vi "COD主界面（列队使用）.vi"() -> (8 "多列列表框":i32(listbox))   [LabVIEW 2016, in "斯坦道CODMn.lvlib"]
uses:
  <vilib>/Analysis/6fits.llb/Curve Fitting Criteria.ctl
  <vilib>/Utility/miscctls.llb/LVPointTypeDef.ctl
  <vilib>/Plasmionique/MB Master/MB_Master_Serial/MB_Master_Serial.lvclass
  D:/Program Files (x86)/National Instruments/LabVIEW 2016/vi.lib/Plasmionique/MB Master/MB_Master/MB_Master.lvclass
  <vilib>/Utility/config.llb/Read Key (Double).vi
  <vilib>/Utility/config.llb/Read Key (Boolean).vi
  <vilib>/Utility/config.llb/Write Key (Double).vi
  <vilib>/Utility/config.llb/Read Key (I32).vi
  <vilib>/Utility/config.llb/Write Key (Boolean).vi
  <vilib>/Utility/config.llb/Write Key (I32).vi
  <vilib>/Waveform/WDTFileIO.llb/Read Waveform from File.vi
  <vilib>/Plasmionique/MB Master/MB Master.lvlib
  <vilib>/ptbypt/NI_PtbyPt.lvlib
  PLC/PLC.lvlib
  <vilib>/Utility/config.llb/NI_LVConfig.lvlib
  <vilib>/Analysis/NI_AALPro.lvlib
panel:
  out "数据时间":string
  out "断电排液标记":bool
  in  "测量模式":T1(ring)
  in  "高切低阈值":dbl
  in  "低切高阈值":dbl
  out "COM":string
  in  "启用5":bool
  in  "校准5":bool
  in  "泵滴定数5":dbl
  in  "浓度5":dbl
  in  "启用4":bool
  in  "校准4":bool
  in  "泵滴定数4":dbl
  in  "浓度4":dbl
  out "波形时间":timestamp
  in  "历史波形":bool
  out "滴定数-ORP值":u16[](array[numeric]) caption="数组"
  in  "关闭 3":bool
  in  "滴定曲线":bool
  out "ORP滴定曲线2":u16[](graph)
  in  "跨度液浓度":dbl
  out "空白测试标记":bool
  out "跨度核查标记":bool
  out "启动选择 2":u16(ring) items=["水样测试", "标样核查", "零点核查", "跨度核查", "空白测试", "加标回收", "平行样", "校零", "校标"]
  in  "量程选择":enum16{"低量程", "高量程", "0-2量程"}(ring)
  in  "手动控制":bool
  in  "选用水样":enum16{"葡萄糖", "草酸钠"}(ring)
  in  "方程系数":cluster{"X^2":dbl, "X":dbl, "b":dbl} {"X^2" format="%#.6g"; "b" format="%#.6g"; "X" format="%#.6g"}
  out "多项式系数1":dbl[](array[numeric]) caption="多项式系数"
  out "XY图":cluster{"X Values":dbl[], "Y Values":dbl[]}[](graph)
  in  "模型":enum32{"线性", "多项式"}(ring)
  out "启动时间":timestamp format="%<%Y/%m/%d %H:%M:%S>T"
  in  "自动切换量程":bool=TRUE
  in  "24H周期设置":bool[](xcontrol)
  in  "关闭 2":bool
  in  "周期设置":bool
  out "文本.文本":string
  out "r^2":dbl format="%.8g"
  out "拟合公式":string
  out "b":dbl format="%#.4g"
  out "K":dbl format="%#.4f"
  out "当前校准":i32
  in  "启用3":bool
  in  "启用2":bool
  in  "启用1":bool
  in  "校准3":bool
  in  "校准2":bool
  in  "校准1":bool
  in  "泵滴定数3":dbl
  in  "泵滴定数2":dbl
  in  "泵滴定数1":dbl
  in  "浓度3":dbl
  in  "浓度2":dbl
  in  "浓度1":dbl
  in  "写入":bool
  out "测量模式数字":i32
  out "零点核查标记":bool
  out "排液故障":bool
  out "进水样超量程":bool
  out "标样核查标记":bool
  out "平行样测量":bool
  out "加标回收测量":bool
  out "质控样测量":bool
  out "待机":bool
  out "校标错误":bool
  out "校零错误":bool
  out "测量错误":bool
  out "草酸钠报警":bool
  out "高锰酸钾报警":bool
  out "加热故障":bool
  out "温控器故障":bool
  out "ORP故障":bool
  out "排液标记":bool
  out "故障标记":bool
  out "校标标记":bool
  out "校零标记":bool
  out "通讯状态":bool
  out "水样测量":bool
  out "读取KB值":bool
  in  "读取":bool
  in  "返回":bool
  in  "校准配置":bool
  in  "修正系数 2":dbl
  in  "浓度 2":dbl
  in  "温度":dbl
  in  "恒温时间":dbl
  in  "基本量程":enum16{"10mg/L", "20mg/L"}(ring)
  in  "水样":dbl
  in  "蒸馏水":dbl
  in  "标液":dbl
  in  "质控样":dbl
  in  "加标回收":dbl
  in  "草酸钠":dbl
  in  "高锰酸钾":dbl
  in  "硫酸":dbl
  in  "零点泵计量数 2":dbl
  in  "标度泵计量数 2":dbl
  out "标度滴定值":dbl
  out "零点滴定值":dbl
  in  "保存":bool
  in  "关闭":bool
  out "测量数据区":T2 {"单位" items=["ug/L", "mg/L", "ppm", "mg/m3", "cm", "ppb", "ug/m3", "%", "nmol/mol", "umol/mol", "MPN/L", "MPN/100ml", "ng/m3", "NTU", "无量纲", "ms/cm", "us/cm", "℃", "mV", "万个/L"]}
  out "仪器时间":timestamp format="%<%Y/%m/%d %H:%M:%S>T"
  out "秒":u16
  out "分":u16
  out "COD浓度（mg/L)":dbl format="%.2g"
  out "进样管":dbl
  out "高锰酸钾":dbl
  out "草酸钠":dbl
  out "硫酸":dbl
  out "ORP显示":dbl
  out "温度":dbl
  out "加热":bool
  out "搅拌":bool
  out "进硫酸":bool
  out "进加标回收样":bool
  out "进质控样":bool
  out "进标液":bool
  out "进蒸馏水":bool
  out "进水样":bool
  out "进草酸钠":bool
  out "进高锰酸钾":bool
  out "定时启动":bool
  in  "启动":bool
  in  "故障清除":bool
  in  "参数配置":bool
  in  "停止":bool
  in  "单步启动":bool
  out "系统时间":timestamp
  in  "时间校准":bool
  in  "枚举":enum16{"读取数据", "写入数据", "读取写入DATABASE", "读取参数"}(ring)
  out "报警簇":T3
  out "Registers":u16[](array[numeric])
  in  "Slave ID":u8=1
  in  "Serial Config":T4={"baud rate (bps)"=115200, "stop bits"=10, "parity"=0, "flow control"=0, "timeout"=1000, "retries"=1} {"stop bits" items=["1.0"=10, "1.5"=15, "2.0"=20]; "flow control" items=["None", "XON/XOFF", "RTS/CTS", "XON/XOFF & RTS/CTS", "DTR/DSR", "XON/XOFF & DTR/DSR"]; "parity" items=["None", "Odd", "Even", "Mark", "Space"]}
  in  "温度 2":dbl
  in  "浓度":dbl
  in  "修正系数":dbl
  in  "标样浓度 2":dbl
  out "模式（受控）":u16
  in  "VISA resource name":refnum<visa-resource-name>="COM4" caption="VISA资源名称"
  # "测量时间："
  # "水样~加标回收"
  # "mV"
  # "℃"
  # "注：遇到加热故障和排液故障时仪器不能正常启动，\n必须排查故障并点击报警清除按钮方可运行。"
  # "mg/L"
  # "校零校标结果"
  # "基本参数设置"
  # "泵计量参数设置"
  # "校零结果："
  # "校零滴定值："
  # "加热恒温温度（℃）："
  # "水样："
  # "高锰酸钾："
  # "校标结果："
  # "标度滴定值："
  # "零点泵计量值："
  # "恒温时间（分钟）："
  # "蒸馏水："
  # "草酸钠："
  # "标度泵计量值："
  # "标准液浓度（mg/L）："
  # "标液："
  # "标样浓度："
  # "硫酸："
  # "修正系数："
  # "质控样："
  # "跨度液浓度："
  # "基本量程（20mg/L可选）："
  # "加标回收样："
  # "是否启用"
  # "泵滴定数"
  # "浓度"
  # "辅\n助\n计\n算\n区"
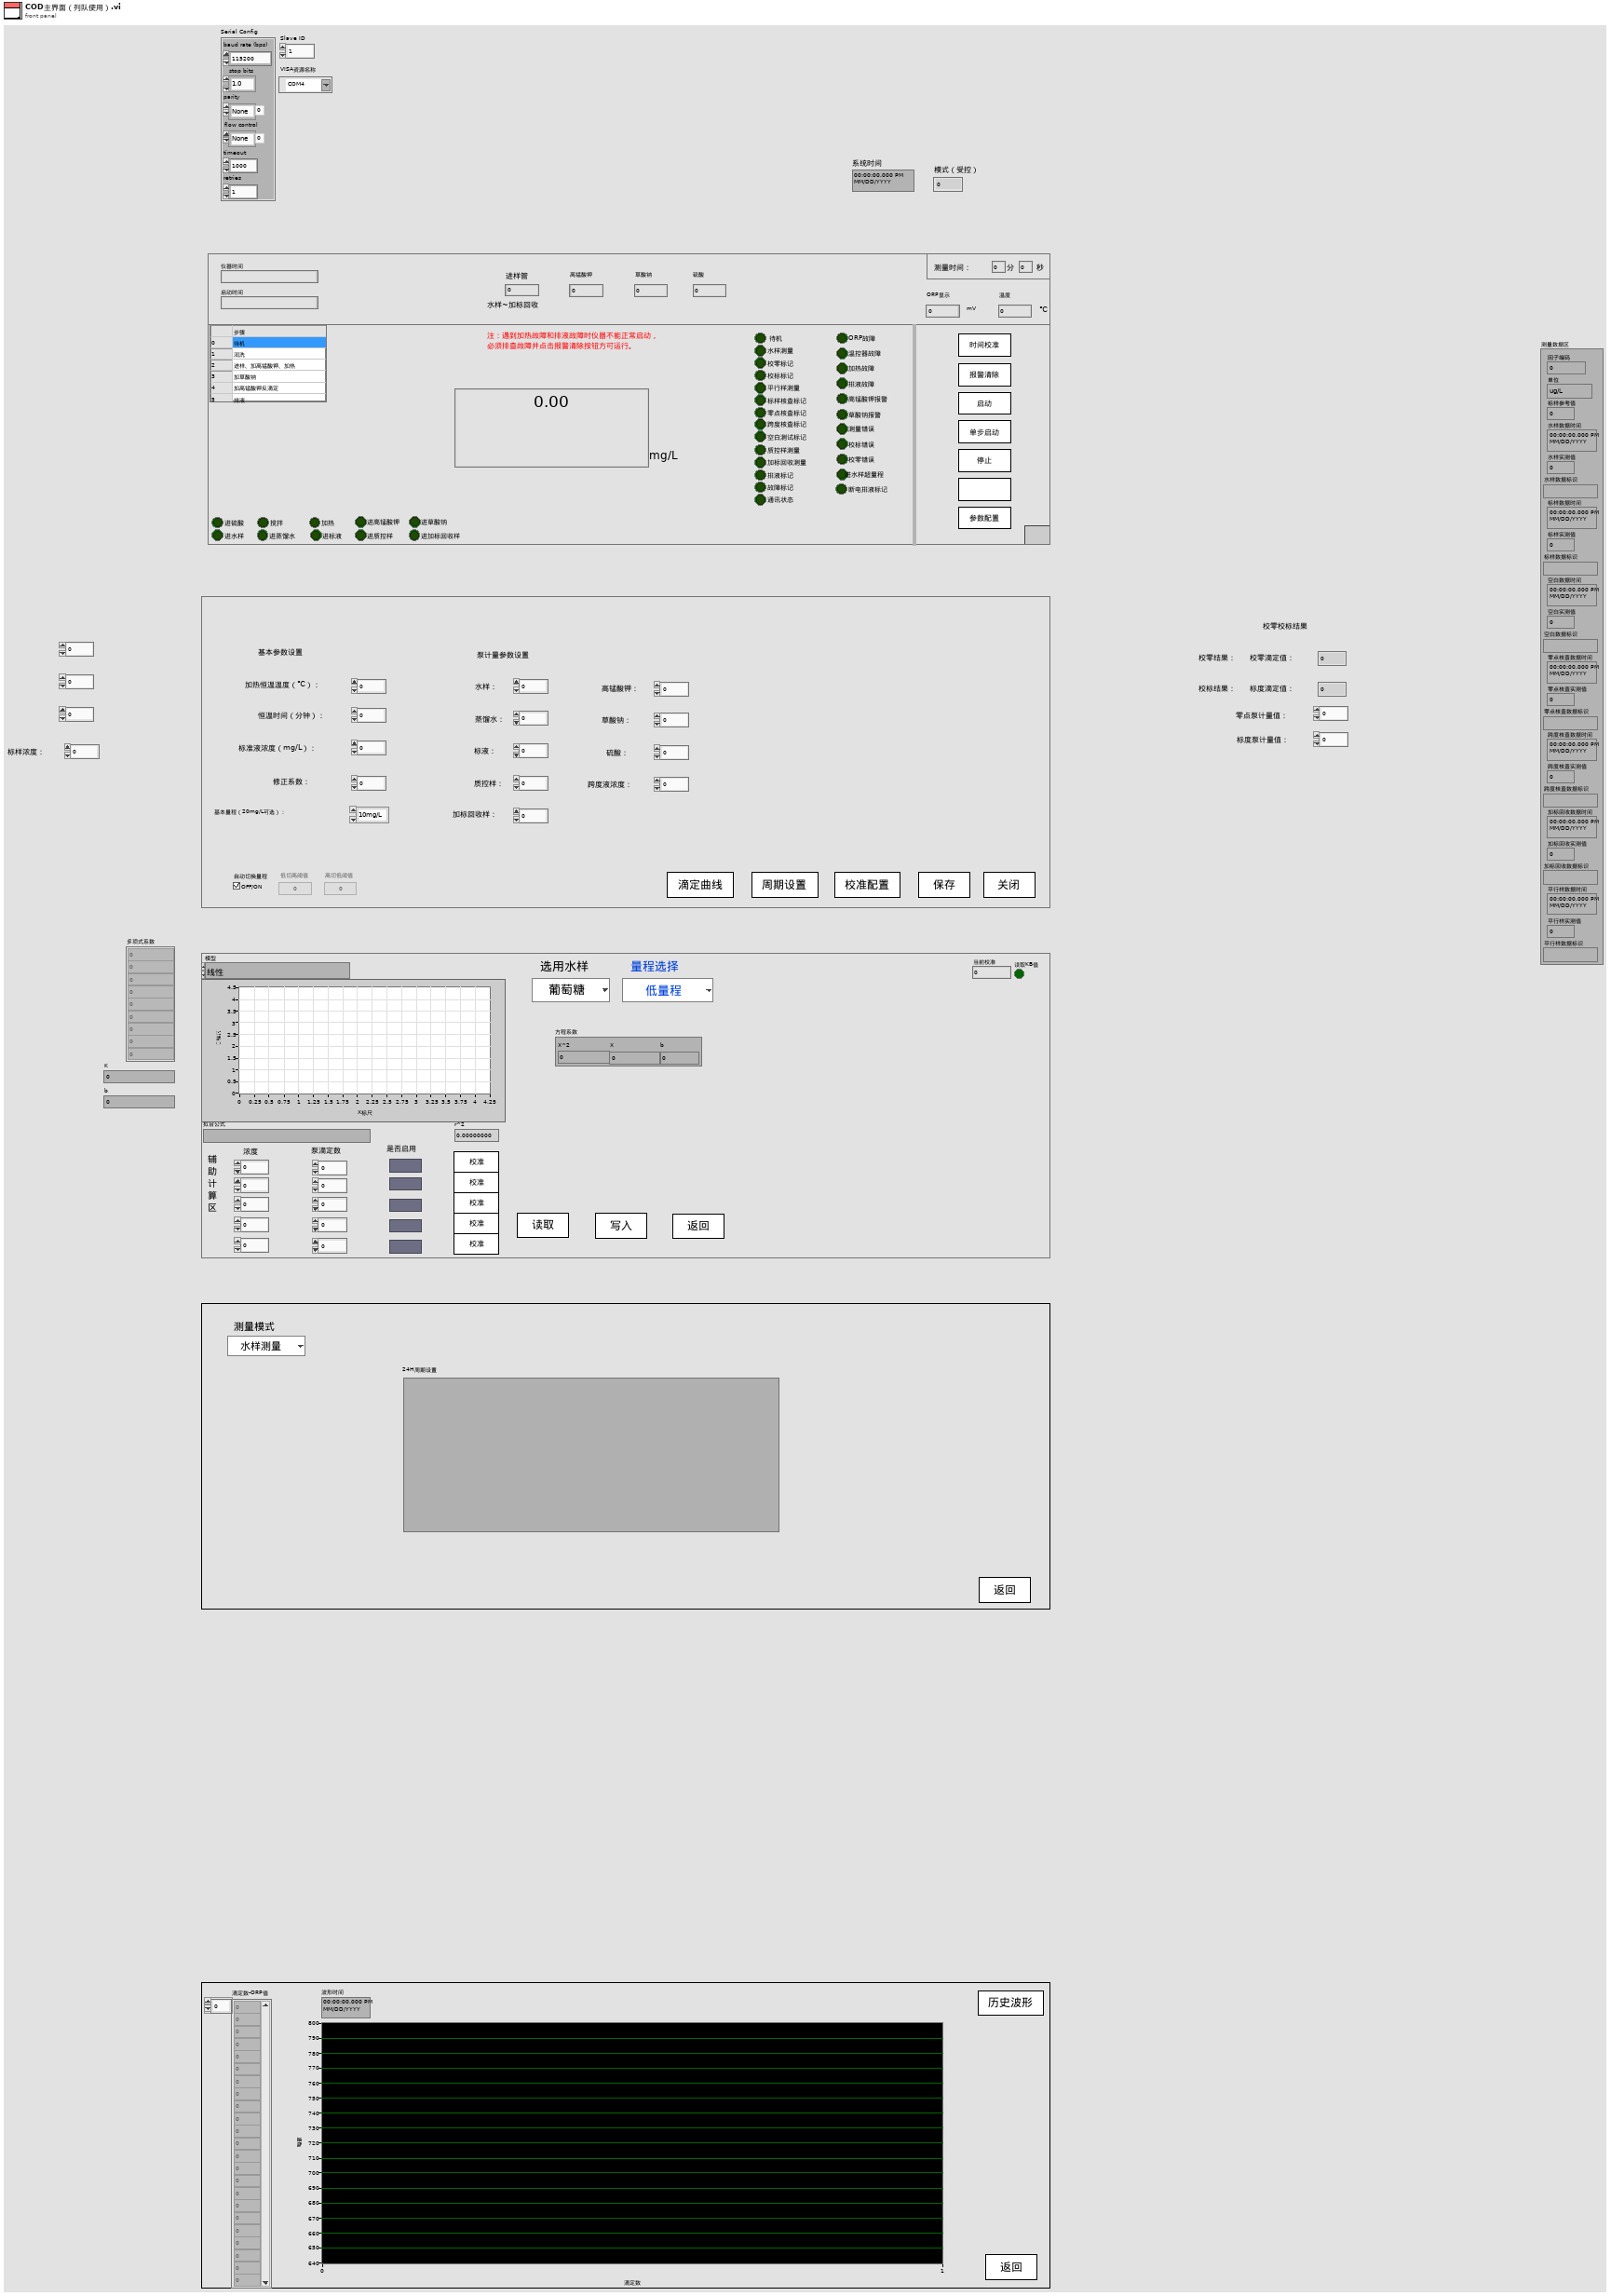
[diagram p1: front panel]
types:
  T1 = enum16{"水样测量", "标样核查", "零点核查", "跨度核查", "空白测试", "加标回收", "平行样", "校零", "校标"}
  T2 = cluster{"因子编码":u32, "单位":u16, "标样参考值":sgl, "水样数据时间":timestamp, "水样实测值":sgl, "水样数据标识":string, "标样数据时间":timestamp, "标样实测值":sgl, "标样数据标识":string, "空白数据时间":timestamp, "空白实测值":sgl, "空白数据标识":string, "零点核查数据时间":timestamp, "零点核查实测值":sgl, "零点核查数据标识":string, "跨度核查数据时间":timestamp, "跨度核查实测值":sgl, "跨度核查数据标识":string, "加标回收数据时间":timestamp, "加标回收实测值":sgl, "加标回收数据标识":string, "平行样数据时间":timestamp, "平行样实测值":sgl, "平行样数据标识":string}
  T3 = cluster{"ORP故障":bool, "温控器故障":bool, "加热故障":bool, "高锰酸钾报警":bool, "草酸钠报警":bool, "测量错误":bool, "校零错误":bool, "校标错误":bool, " 进水样超量程":bool, "排液阀故障":bool}
  T4 = cluster{"baud rate (bps)":u32, "stop bits":u16, "parity":u16, "flow control":u16, "timeout":u32, "retries":i32}
  T5 = cluster{"starting address":u16, "number of holding registers":u16}
  T6 = cluster{"测量模式":enum16{"水样测量", "标样核查", "零点核查", "跨度核查", "空白测试", "加标回收", "平行样", "校零", "校标"}}
  T7 = cluster{"仪器测试类型":enum16{"水样测试", "标样核查", "空白测试", "跨度核查"}, "周期设置类型":enum16{"定点启动", "间隔启动"}, "定时功能启用":bool, "定时间隔":dbl, "24H周期设置":bool[]}
  T8 = typedef "LVDateTimeRec.ctl" = cluster{"秒数的小数部分":dbl, "秒":i32, "分":i32, "时":i32, "日":i32, "月":i32, "年":i32, "天数（周）":i32, "天数（年）":i32, "DST":i32}
  T9 = typedef "LVPointTypeDef.ctl" = cluster{"Horizontal":i16, "Vertical":i16}
  T10 = typedef "NI_LVConfig.lvlib/Config Data RefNum.ctl" = refnum<k1>
  T11 = enum8{"Enabled", "Disabled", "Disabled and Grayed Out"}
  T12 = cluster{"时间标识":timestamp, "参数":string, "日志信息":string, "流程参数":string}
  T13 = cluster{"时间标识":timestamp, "设备":string, "日志信息":string}
  T14 = typedef "NI_AALPro.lvlib/Curve Fitting Criteria.ctl" = u16
  T15 = cluster{"时间标识":timestamp, "设备":string, "日志信息":string, "流程参数":string}
  T16 = cluster{"时间":timestamp, "测量模式":string, "数据类型":string, "检测值":sgl, "单位":string, "数据标识":string, "因子编码":string, "标样参考值":sgl, "ORP-A":sgl, "ORP-B":sgl, "ORP-K":sgl, "COD滴定值":sgl, "高锰酸钾滴定数":sgl, "温度":sgl}
  T17 = cluster{"数组 2[0]":sgl, "数组 2[1]":sgl, "数组 2[2]":sgl, "数组 2[3]":sgl, "数组 2[4]":sgl, "数组 2[5]":sgl, "数组 2[6]":sgl, "数组 2[7]":sgl, "数组 2[8]":sgl}
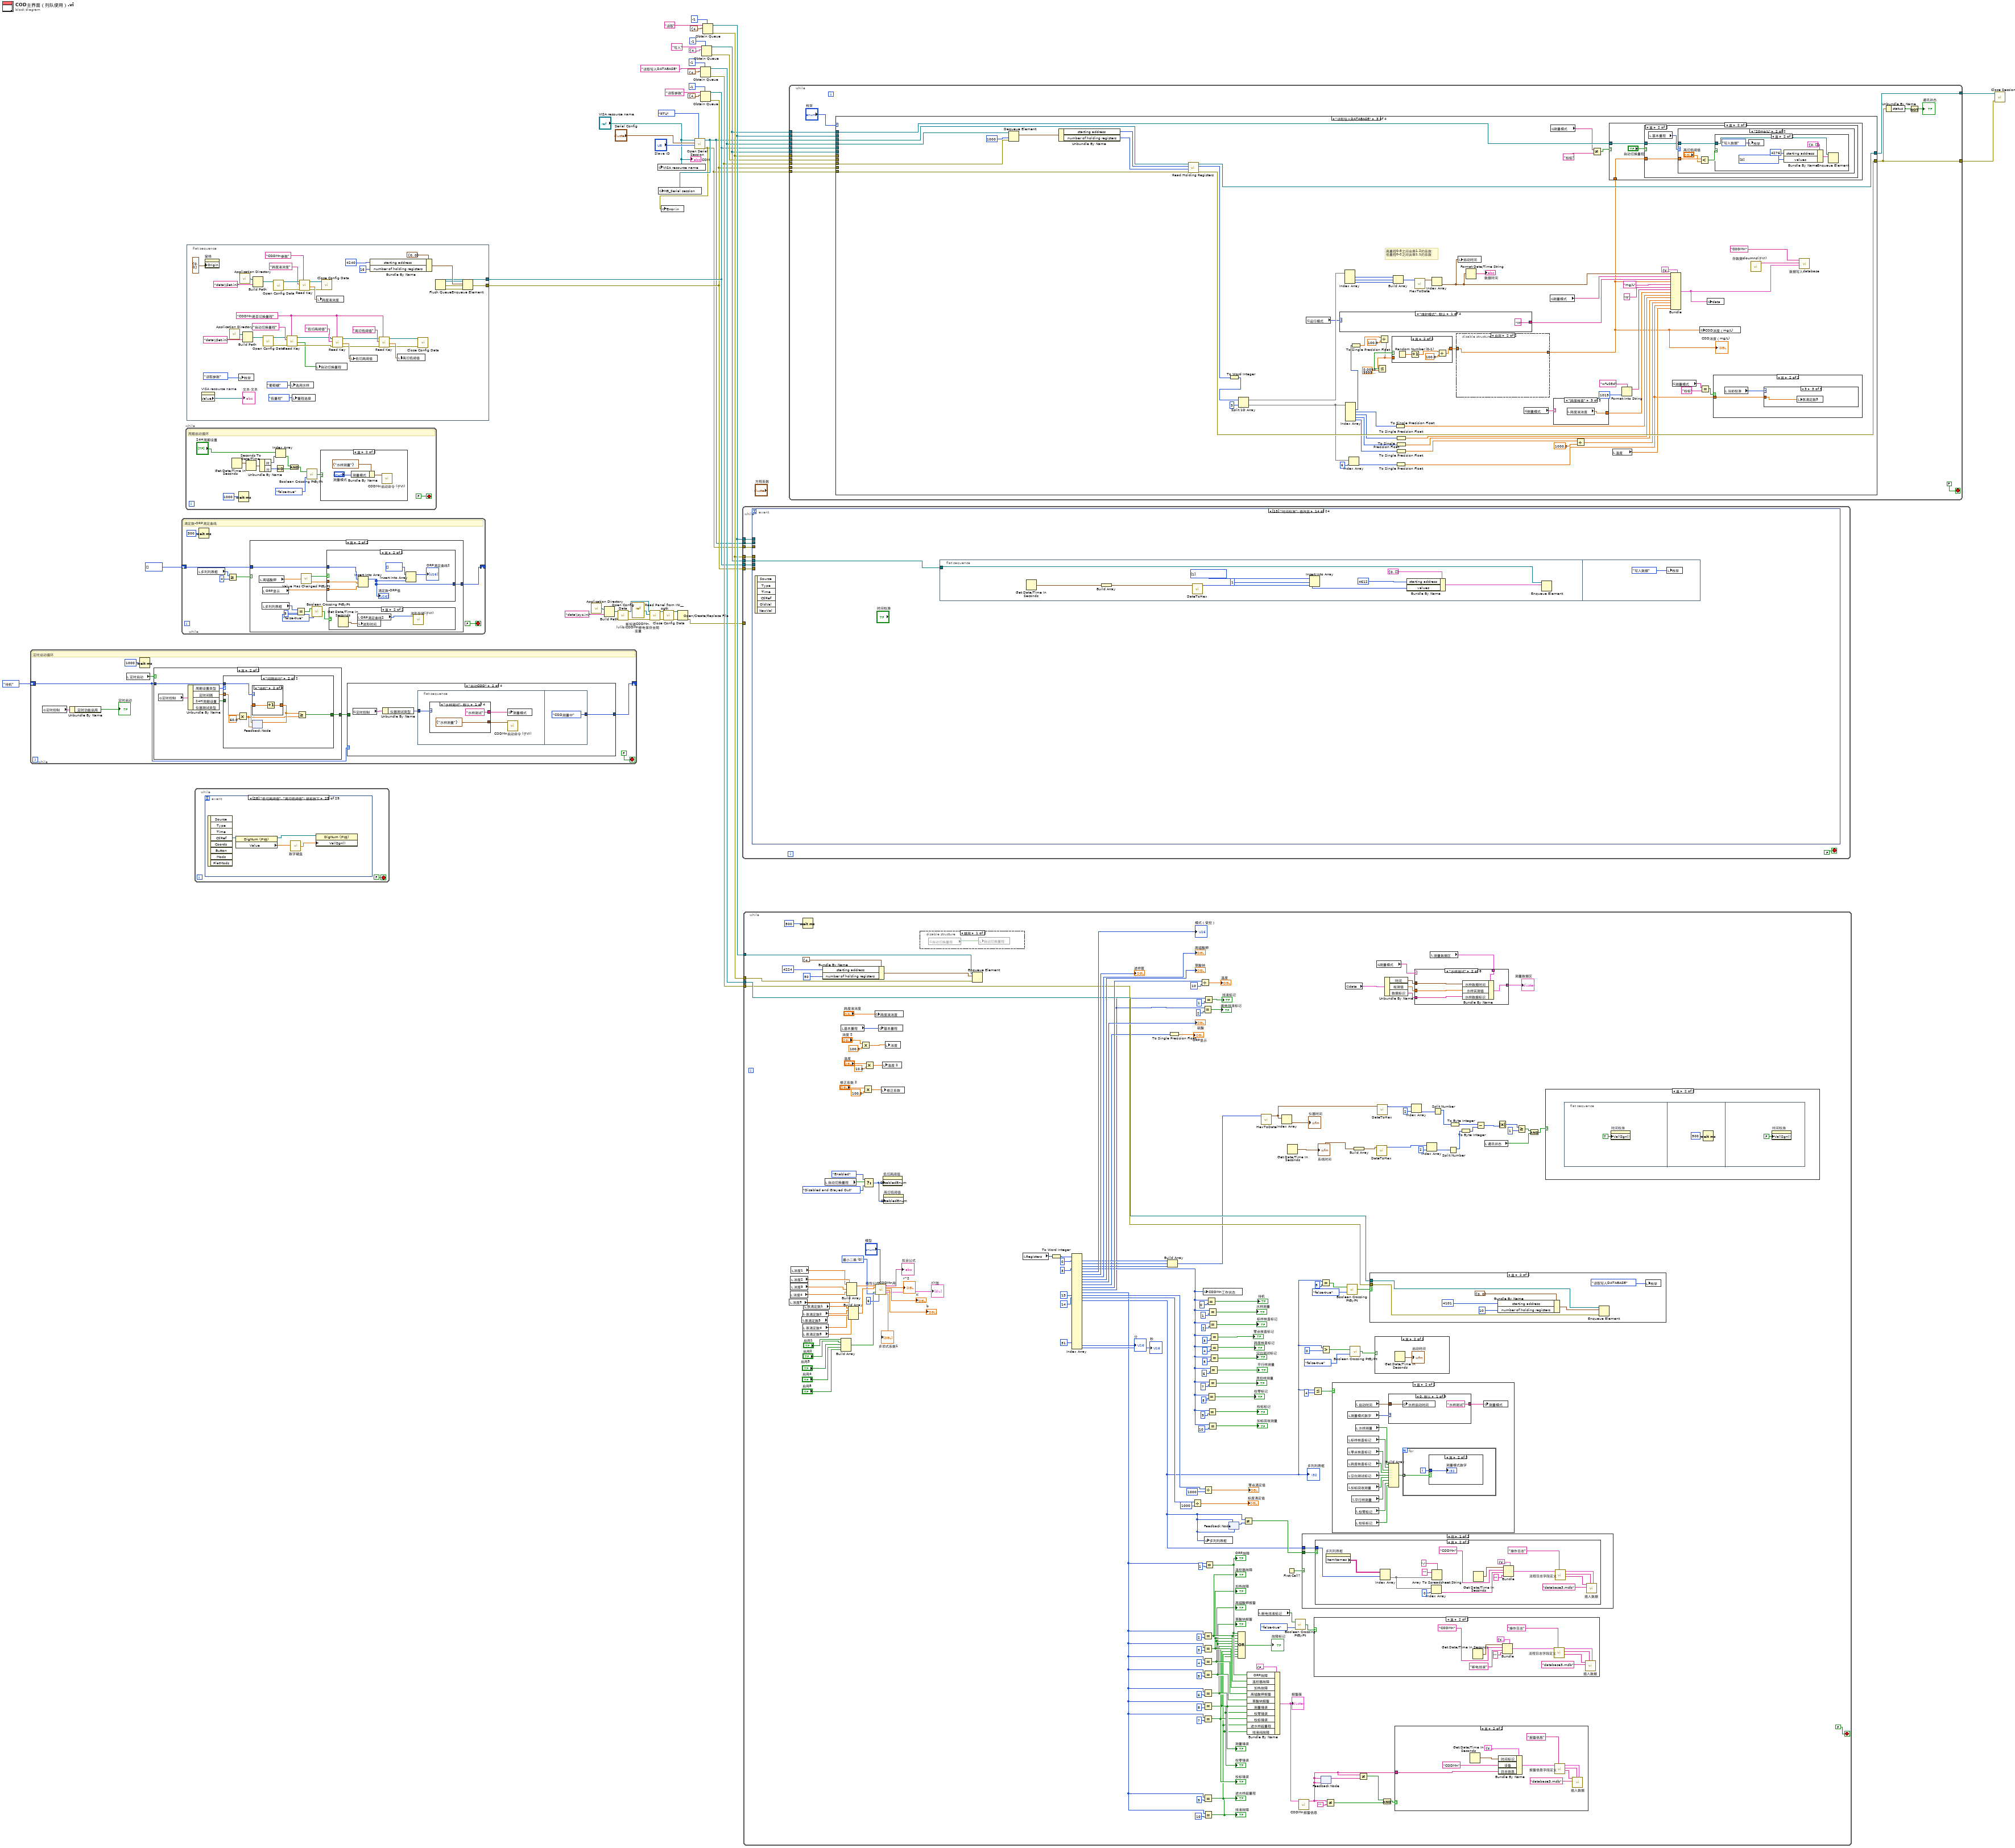
[diagram p0: block diagram]
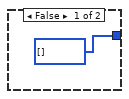
[diagram p2: hidden frame]
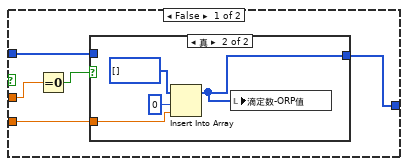
[diagram p4: hidden frame]
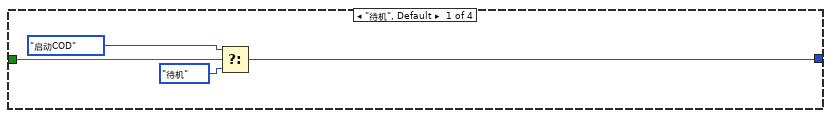
[diagram p7: hidden frame]
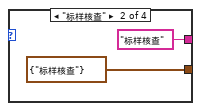
[diagram p8: hidden frame]
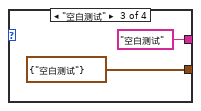
[diagram p9: hidden frame]
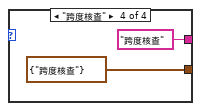
[diagram p10: hidden frame]
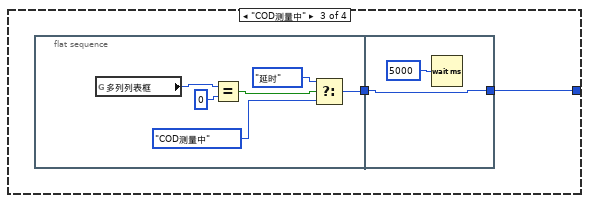
[diagram p11: hidden frame]
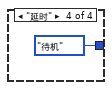
[diagram p12: hidden frame]
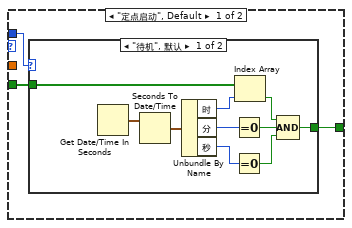
[diagram p14: hidden frame]
diagram:
  n1 = while {
    shift-right: [w47] -> _
    shift-left: enum16{"待机", "启动COD", "COD测量中", "延时"}."待机" -> [w46]
    stop <- FALSE stop-if-true
    # "定时启动循环"
    n2 = global read "CODMn断电保存全局变量.vi" "定时控制"() -> (w43:T7)
    n3 = Unbundle By Name(w43) -> ("定时功能启用"=→"定时启动":bool)
    n4 = local read "定时启动"() -> (w44:bool)
    n5 = Wait (ms)(milliseconds to wait=u32 1000 ("等待时间（毫秒）")) -> ()  [unwired: 1 out]
    n6 = case shown="真" w44 {
      tunnel: w46 -> [_ w82]
      tunnel: [_ w81] -> w45
      frame False {
      }
      frame True {
        n7 = global read "CODMn断电保存全局变量.vi" "定时控制"() -> (w80:T7)
        n8 = Unbundle By Name(w80) -> ("周期设置类型"=w83:enum16{"定点启动", "间隔启动"}, "定时间隔"=w84:dbl, "24H周期设置"=w85:bool[])  [unwired: 1 out]
        n9 = case shown="\"间隔启动\"" w83 {
          tunnel: w84 -> [_ w102]
          tunnel: w85 -> [w88 _]
          tunnel: w82 -> [w86 w105]
          tunnel: [w87 w100] -> w81
          frame "定点启动", Default {
            n10 = case shown="\"待机\", 默认" w86 {
              tunnel: w88 -> [w96 _]
              tunnel: [w89 _] -> w87
              frame "待机", Default {
                n11 = Get Date/Time In Seconds() -> (seconds since 1Jan1904=w98:timestamp)
                n12 = Seconds To Date/Time(time stamp (now)=w98) -> (date time rec=w97:T8)  [unwired: 1 in]
                n13 = Unbundle By Name(w97) -> ("时"=w95:i32, "分"=w93:i32, "秒"=w94:i32)
                n14 = Equal To 0?(x=w93) -> (x = 0?=w91:bool)
                n15 = Equal To 0?(x=w94) -> (x = 0?=w90:bool)
                n16 = Index Array(array=w96, index=w95) -> (element=w92:bool)
                n17 = Compound Arithmetic op=AND ("复合运算")(w92, w91, w90) -> (w89:bool)
              }
              frame "启动COD" {
              }
            }
          }
          frame "间隔启动" {
            n18 = Multiply(x=w102, y=60.0) -> (x*y=w99:dbl)
            n19 = feedback #1(w99) -> (w104:dbl)
            n20 = case shown="\"待机\"" w105 {
              tunnel: w104 -> [_ w107]
              tunnel: [_ w106] -> w103
              frame Default {
              }
              frame "待机" {
                n21 = Increment(x=w107) -> (x+1=w106:dbl)
              }
            }
            n22 = feedback-in #1(w103) -> ()
            n23 = Greater Or Equal?(x=w103, y=w99) -> (x >= y?=w100:bool)
          }
        }
      }
    }
    n24 = case shown="\"启动COD\"" w46 {
      tunnel: [w50 w56 w70 enum16{"待机", "启动COD", "COD测量中", "延时"}."待机"] -> w47
      tunnel: w45 -> [w53 _ _ _]
      frame "待机", Default {
        n25 = Select(t=enum16{"待机", "启动COD", "COD测量中", "延时"}."启动COD", s=w53, f=enum16{"待机", "启动COD", "COD测量中", "延时"}."待机") -> (s? t:f=w50:enum16{"待机", "启动COD", "COD测量中", "延时"})
      }
      frame "启动COD" {
        n26 = global read "CODMn断电保存全局变量.vi" "定时控制"() -> (w54:T7)
        n27 = Unbundle By Name(w54) -> ("仪器测试类型"=w55:enum16{"水样测试", "标样核查", "空白测试", "跨度核查"})
        n28 = flat-sequence {
          tunnel: w55 -> [w59]
          tunnel: [enum16{"待机", "启动COD", "COD测量中", "延时"}."COD测量中"] -> w56
          frame #0 {
            n29 = case shown="\"水样测试\", 默认" w59 {
              tunnel: [T6 {"测量模式"=enum."水样测量"} ("启动测量模式") T6 {"测量模式"=enum."标样核查"} ("启动测量模式") T6 {"测量模式"=enum."空白测试"} ("启动测量模式") T6 {"测量模式"=enum."跨度核查"} ("启动测量模式")] -> w58
              tunnel: ["水样测试" ("测量模式") "标样核查" ("测量模式") "空白测试" ("测量模式") "跨度核查" ("测量模式")] -> w57
              frame "水样测试", Default {
              }
              frame "标样核查" {
              }
              frame "空白测试" {
              }
              frame "跨度核查" {
              }
            }
            n30 = global write "COD测量模式全局.vi" "测量模式"(w57) -> ()
            n31 = call "CODMn启动命令 (子VI).vi"("启动测量模式"=w58) -> ()  [unwired: 11 in]
          }
          frame #1 {
          }
        }
      }
      frame "COD测量中" {
        n32 = flat-sequence {
          tunnel: [w71] -> w69
          tunnel: [w78] -> w70
          tunnel: w69 -> [w78]
          frame #0 {
            n33 = global read "运行时序全局变量.vi" "多列列表框"() -> (w76:i32)
            n34 = Equal?(x=w76, y=0) -> (x = y?=w74:bool)
            n35 = Select(t=enum16{"待机", "启动COD", "COD测量中", "延时"}."延时", s=w74, f=enum16{"待机", "启动COD", "COD测量中", "延时"}."COD测量中") -> (s? t:f=w71:enum16{"待机", "启动COD", "COD测量中", "延时"})
          }
          frame #1 {
            n36 = Wait (ms)(milliseconds to wait=u32 5000 ("等待时间（毫秒）")) -> ()  [unwired: 1 out]
          }
        }
      }
      frame "延时" {
      }
    }
  }
  n37 = while {
    shift-right: [w111] -> _
    shift-left: u16[] [] ("ORP滴定曲线") -> [w112]
    stop <- FALSE stop-if-true
    # "滴定数-ORP滴定曲线"
    n38 = local read "多列列表框"() -> (w110:i32)
    n39 = Wait (ms)(milliseconds to wait=u32 300 ("等待时间（毫秒）")) -> ()  [unwired: 1 out]
    n40 = Greater Or Equal?(x=w110, y=4) -> (x >= y?=w108:bool)
    n41 = case shown="真" w108 {
      tunnel: w112 -> [_ w126]
      tunnel: [u16[] [] ("ORP滴定曲线") w125] -> w111
      frame False {
      }
      frame True {
        n42 = local read "高锰酸钾"() -> (w122:dbl)
        n43 = local read "多列列表框"() -> (w120:i32)
        n44 = local read "ORP显示"() -> (w121:dbl)
        n45 = Equal?(x=w120, y=5) -> (x = y?=w118:bool)
        n46 = call <vilib>:"Value Has Changed PtByPt.vi"("input data point"=w122) -> ("has changed"=w124:bool, "output data point"=w123:dbl)  [unwired: 1 in]
        n47 = call <vilib>:"Boolean Crossing PtByPt.vi"("direction"=enum16{"either", "false-true", "true-false"}."false-true", "input"=w118) -> ("crossing"=w116:bool)  [unwired: 1 in]
        n48 = case shown="真" w124 {
          tunnel: w126 -> [w132 w142]
          tunnel: [w131 w141] -> w125
          tunnel: w123 -> [w133 w140]
          tunnel: w121 -> [w129 w139]
          frame False {
            n49 = Equal To 0?(x=w133) -> (x = 0?=w130:bool)
            n50 = case shown="真" w130 {
              tunnel: [w134 w137] -> w131
              tunnel: w132 -> [w134 _]
              tunnel: w129 -> [_ w136]
              frame False {
              }
              frame True {
                n51 = Insert Into Array(array=u16[] [] ("ORP滴定曲线"), index=0 ("索引"), new element=w136) -> (w137:u16[])
                n52 = local write "滴定数-ORP值"(w137) -> ()
              }
            }
          }
          frame True {
            n53 = Insert Into Array(array=w142, index=w140, new element=w139) -> (w141:u16[])
            "滴定数-ORP值" <- w141
            n54 = Insert Into Array(array=u16[] [] ("ORP滴定曲线"), new element=w141) -> (→"ORP滴定曲线2":u16[])  [unwired: 1 in]
          }
        }
        n55 = case shown="真" w116 {
          frame False {
          }
          frame True {
            n56 = Get Date/Time In Seconds() -> (seconds since 1Jan1904=w127:timestamp)
            n57 = local read "ORP滴定曲线2"() -> (w128:u16[])
            n58 = local write "波形时间"(w127) -> ()
            n59 = call "波形存储(子VI).vi"("ORP滴定曲线"=w128) -> ()  [unwired: 11 in]
          }
        }
      }
    }
  }
  n60 = while "While循环" {
    stop <- FALSE stop-if-true
    # "周期启动循环"
    n61 = Get Date/Time In Seconds() -> (seconds since 1Jan1904=w156:timestamp)
    n62 = Wait (ms)(milliseconds to wait=u32 1000 ("等待时间（毫秒）")) -> ()  [unwired: 1 out]
    n63 = Seconds To Date/Time(time stamp (now)=w156) -> (date time rec=w155:T8)  [unwired: 1 in]
    n64 = Unbundle By Name(w155) -> ("时"=w152:i32, "分"=w154:i32)
    n65 = Equal To 0?(x=w154) -> (x = 0?=w153:bool)
    n66 = Index Array(array="24H周期设置", index=w152) -> (element=w151:bool)
    n67 = And(x=w151, y=w153) -> (x .and. y?=w149:bool)
    n68 = call <vilib>:"Boolean Crossing PtByPt.vi"("direction"=enum16{"either", "false-true", "true-false"}."false-true", "input"=w149) -> ("crossing"=w148:bool)  [unwired: 1 in]
    n69 = case shown="真" w148 {
      frame False {
      }
      frame True {
        n70 = Bundle By Name(cluster=T6 {"测量模式"=enum."水样测量"} ("启动测量模式"), "测量模式"="测量模式") -> (w158:T6)
        n71 = call "CODMn启动命令 (子VI).vi"("启动测量模式"=w158) -> ()  [unwired: 11 in]
      }
    }
  }
  n72 = flat-sequence {
    tunnel: w15 -> [w182]
    tunnel: w14 -> [w181]
    frame #0 {
      w174 = "CODMn是否切换量程" ("key")
      n73 = property on="VISA resource name" class="VISAName"() -> ("Value"=→"文本.文本":refnum<visa-resource-name>)  [unwired: 2 in, 2 out]
      n74 = property on="窗格" class="Pane"("Origin"=T9 {"Horizontal"=0, "Vertical"=0} ("原点")) -> ()  [unwired: 2 in, 2 out]
      n75 = call <vilib>:"Application Directory.vi"() -> ("Application Directory"=w165:path)
      n76 = local write "枚举"(enum16{"读取数据", "写入数据", "读取写入DATABASE", "读取参数"}."读取参数" ("枚举")) -> ()
      n77 = call <vilib>:"Application Directory.vi"() -> ("Application Directory"=w190:path)
      n78 = Build Path(base path=w165, name or relative path="data\\Set.ini" ("名称或相对路径")) -> (appended path=w167:path)
      n79 = Build Path(base path=w190, name or relative path="data\\Set.ini" ("名称或相对路径")) -> (appended path=w192:path)
      n80 = call <vilib>:"Open Config Data.vi"("configuration file path"=w167) -> ("error out"=w164:errorcluster, "refnum"=w163:T10)  [unwired: 8 in, 1 out]
      n81 = call <vilib>:"Open Config Data.vi"("configuration file path"=w192) -> ("error out"=w196:errorcluster, "refnum"=w195:T10)  [unwired: 8 in, 1 out]
      n82 = call-poly <vilib>:"Read Key.vi"("section"=w174, "error in (no error)"=w164, "key"="自动切换量程", "refnum"=w163) -> ("error out"=w171:errorcluster, "value"=w169:bool, "refnum out"=w170:T10)  [unwired: 4 in, 1 out]
      n83 = local write "选用水样"(enum16{"葡萄糖", "草酸钠"}."葡萄糖" ("选用水样")) -> ()
      n84 = local write "量程选择"(enum16{"低量程", "高量程", "0-2量程"}."低量程" ("量程选择")) -> ()
      n85 = call-poly <vilib>:"Read Key.vi"("section"="CODMn参数" ("key"), "error in (no error)"=w196, "key"="跨度液浓度", "refnum"=w195) -> ("error out"=w198:errorcluster, "value"=w199:dbl, "refnum out"=w197:T10)  [unwired: 4 in, 1 out]
      n86 = local write "自动切换量程"(w169) -> ()
      n87 = local write "跨度液浓度"(w199) -> ()
      n88 = call <vilib>:"Close Config Data.vi"("error in (no error)"=w198, "refnum"=w197) -> ()  [unwired: 8 in, 2 out]
      n89 = call-poly <vilib>:"Read Key.vi"("section"=w174, "error in (no error)"=w171, "key"="低切高阈值", "refnum"=w170) -> ("error out"=w173:errorcluster, "value"=w179:dbl, "refnum out"=w172:T10)  [unwired: 4 in, 1 out]
      n90 = local write "低切高阈值"(w179) -> ()
      n91 = Bundle By Name(cluster=T5 {"starting address"=0, "number of holding registers"=0}, "starting address"=u16 4240, "number of holding registers"=u16 16) -> (w189:T5)
      n92 = call-poly <vilib>:"Read Key.vi"("section"=w174, "error in (no error)"=w173, "key"="高切低阈值", "refnum"=w172) -> ("error out"=w176:errorcluster, "value"=w180:dbl, "refnum out"=w175:T10)  [unwired: 4 in, 1 out]
      n93 = local write "高切低阈值"(w180) -> ()
      n94 = call <vilib>:"Close Config Data.vi"("error in (no error)"=w176, "refnum"=w175) -> ()  [unwired: 8 in, 2 out]
      n95 = Flush Queue(queue=w182, error in (no error)=w181) -> (queue out=w185:refnum<queue>, error out=w184:errorcluster)  [unwired: 1 out]
      n96 = Enqueue Element(queue=w185, element=w189, error in (no error)=w184) -> ()  [unwired: 1 in, 3 out]
    }
  }
  n97 = while {
    stop <- FALSE stop-if-true
    n98 = event shown="[28] \"低切高阈值\", \"高切低阈值\": 鼠标按下" {
      selector: _ -> [_ _ _ _ _ _ _ _ _ _ _ _ _ _ _ _ _ _ _ _ _ _ _ _ _ _ _ _ _]
      dyn-events: _ -> [_ _ _ _ _ _ _ _ _ _ _ _ _ _ _ _ _ _ _ _ _ _ _ _ _ _ _ _ _]
      timeout: _ -> [_ _ _ _ _ _ _ _ _ _ _ _ _ _ _ _ _ _ _ _ _ _ _ _ _ _ _ _ _]
      event Timeout {
        n99 = event-data() -> ()  [unwired: 1 in, 3 out]
      }
      event "温度": Mouse Down {
        n100 = event-data() -> ()  [unwired: 1 in, 8 out]
        n101 = local read "温度"() -> (w203:dbl)
        n102 = call "数字键盘.vi"("OldNumber"=w203) -> ("NewNumber"=w202:sgl)
        n103 = local write "温度"(w202) -> ()
      }
      event "恒温时间": Mouse Down {
        n104 = event-data() -> ()  [unwired: 1 in, 8 out]
        n105 = local read "恒温时间"() -> (w204:dbl)
        n106 = call "数字键盘.vi"("OldNumber"=w204) -> ("NewNumber"=w205:sgl)
        n107 = local write "恒温时间"(w205) -> ()
      }
      event "浓度 2": Mouse Down {
        n108 = event-data() -> ()  [unwired: 1 in, 8 out]
        n109 = local read "浓度 2"() -> (w207:dbl)
        n110 = call "数字键盘.vi"("OldNumber"=w207) -> ("NewNumber"=w206:sgl)
        n111 = local write "浓度 2"(w206) -> ()
      }
      event "修正系数 2": Mouse Down {
        n112 = event-data() -> ()  [unwired: 1 in, 8 out]
        n113 = local read "修正系数 2"() -> (w208:dbl)
        n114 = call "数字键盘.vi"("OldNumber"=w208) -> ("NewNumber"=w209:sgl)
        n115 = local write "修正系数 2"(w209) -> ()
      }
      event "水样": Mouse Down {
        n116 = event-data() -> ()  [unwired: 1 in, 8 out]
        n117 = local read "水样"() -> (w210:dbl)
        n118 = call "数字键盘.vi"("OldNumber"=w210) -> ("NewNumber"=w211:sgl)
        n119 = local write "水样"(w211) -> ()
      }
      event "蒸馏水": Mouse Down {
        n120 = event-data() -> ()  [unwired: 1 in, 8 out]
        n121 = local read "蒸馏水"() -> (w212:dbl)
        n122 = call "数字键盘.vi"("OldNumber"=w212) -> ("NewNumber"=w213:sgl)
        n123 = local write "蒸馏水"(w213) -> ()
      }
      event "标液": Mouse Down {
        n124 = event-data() -> ()  [unwired: 1 in, 8 out]
        n125 = local read "标液"() -> (w214:dbl)
        n126 = call "数字键盘.vi"("OldNumber"=w214) -> ("NewNumber"=w215:sgl)
        n127 = local write "标液"(w215) -> ()
      }
      event "质控样": Mouse Down {
        n128 = event-data() -> ()  [unwired: 1 in, 8 out]
        n129 = local read "质控样"() -> (w216:dbl)
        n130 = call "数字键盘.vi"("OldNumber"=w216) -> ("NewNumber"=w217:sgl)
        n131 = local write "质控样"(w217) -> ()
      }
      event "加标回收": Mouse Down {
        n132 = event-data() -> ()  [unwired: 1 in, 8 out]
        n133 = local read "加标回收"() -> (w218:dbl)
        n134 = call "数字键盘.vi"("OldNumber"=w218) -> ("NewNumber"=w219:sgl)
        n135 = local write "加标回收"(w219) -> ()
      }
      event "草酸钠": Mouse Down {
        n136 = event-data() -> ()  [unwired: 1 in, 8 out]
        n137 = local read "草酸钠"() -> (w220:dbl)
        n138 = call "数字键盘.vi"("OldNumber"=w220) -> ("NewNumber"=w221:sgl)
        n139 = local write "草酸钠"(w221) -> ()
      }
      event "高锰酸钾": Mouse Down {
        n140 = event-data() -> ()  [unwired: 1 in, 8 out]
        n141 = local read "高锰酸钾"() -> (w222:dbl)
        n142 = call "数字键盘.vi"("OldNumber"=w222) -> ("NewNumber"=w223:sgl)
        n143 = local write "高锰酸钾"(w223) -> ()
      }
      event "硫酸": Mouse Down {
        n144 = event-data() -> ()  [unwired: 1 in, 8 out]
        n145 = local read "硫酸"() -> (w224:dbl)
        n146 = call "数字键盘.vi"("OldNumber"=w224) -> ("NewNumber"=w225:sgl)
        n147 = local write "硫酸"(w225) -> ()
      }
      event "零点泵计量数 2": Mouse Down {
        n148 = event-data() -> ()  [unwired: 1 in, 8 out]
        n149 = local read "零点泵计量数 2"() -> (w226:dbl)
        n150 = call "数字键盘.vi"("OldNumber"=w226) -> ("NewNumber"=w227:sgl)
        n151 = local write "零点泵计量数 2"(w227) -> ()
      }
      event "标度泵计量数 2": Mouse Down {
        n152 = event-data() -> ()  [unwired: 1 in, 8 out]
        n153 = local read "标度泵计量数 2"() -> (w228:dbl)
        n154 = call "数字键盘.vi"("OldNumber"=w228) -> ("NewNumber"=w229:sgl)
        n155 = local write "标度泵计量数 2"(w229) -> ()
      }
      event "标样浓度 2": Mouse Down {
        n156 = event-data() -> ()  [unwired: 1 in, 8 out]
        n157 = local read "标样浓度 2"() -> (w230:dbl)
        n158 = call "数字键盘.vi"("OldNumber"=w230) -> ("NewNumber"=w231:sgl)
        n159 = local write "标样浓度 2"(w231) -> ()
      }
      event "浓度1": Mouse Down {
        n160 = event-data() -> ()  [unwired: 1 in, 8 out]
        n161 = local read "浓度1"() -> (w233:dbl)
        n162 = call "数字键盘.vi"("OldNumber"=w233) -> ("NewNumber"=w232:sgl)
        n163 = property on="浓度1" class="DigNum (严格)"("Val(Sgnl)"=w232) -> ()  [unwired: 2 in, 2 out]
      }
      event "浓度2": Mouse Down {
        n164 = event-data() -> ()  [unwired: 1 in, 8 out]
        n165 = local read "浓度2"() -> (w235:dbl)
        n166 = call "数字键盘.vi"("OldNumber"=w235) -> ("NewNumber"=w234:sgl)
        n167 = property on="浓度2" class="DigNum (严格)"("Val(Sgnl)"=w234) -> ()  [unwired: 2 in, 2 out]
      }
      event "浓度3": Mouse Down {
        n168 = event-data() -> ()  [unwired: 1 in, 8 out]
        n169 = local read "浓度3"() -> (w237:dbl)
        n170 = call "数字键盘.vi"("OldNumber"=w237) -> ("NewNumber"=w236:sgl)
        n171 = property on="浓度3" class="DigNum (严格)"("Val(Sgnl)"=w236) -> ()  [unwired: 2 in, 2 out]
      }
      event "浓度4": Mouse Down {
        n172 = event-data() -> ()  [unwired: 1 in, 8 out]
        n173 = local read "浓度4"() -> (w239:dbl)
        n174 = call "数字键盘.vi"("OldNumber"=w239) -> ("NewNumber"=w238:sgl)
        n175 = property on="浓度4" class="DigNum (严格)"("Val(Sgnl)"=w238) -> ()  [unwired: 2 in, 2 out]
      }
      event "浓度5": Mouse Down {
        n176 = event-data() -> ()  [unwired: 1 in, 8 out]
        n177 = local read "浓度5"() -> (w241:dbl)
        n178 = call "数字键盘.vi"("OldNumber"=w241) -> ("NewNumber"=w240:sgl)
        n179 = property on="浓度5" class="DigNum (严格)"("Val(Sgnl)"=w240) -> ()  [unwired: 2 in, 2 out]
      }
      event "跨度液浓度": Mouse Down {
        n180 = event-data() -> ()  [unwired: 1 in, 8 out]
        n181 = local read "跨度液浓度"() -> (w243:dbl)
        n182 = call "数字键盘.vi"("OldNumber"=w243) -> ("NewNumber"=w242:sgl)
        n183 = property on="跨度液浓度" class="DigNum (严格)"("Val(Sgnl)"=w242) -> ()  [unwired: 2 in, 2 out]
      }
      event "跨度液浓度": Value Change {
        n184 = event-data() -> ()  [unwired: 1 in, 6 out]
        n185 = call <vilib>:"Application Directory.vi"() -> ("Application Directory"=w247:path)
        n186 = Build Path(base path=w247, name or relative path="data\\Set.ini" ("名称或相对路径")) -> (appended path=w249:path)
        n187 = local read "跨度液浓度"() -> (w244:dbl)
        n188 = call <vilib>:"Open Config Data.vi"("configuration file path"=w249) -> ("error out"=w251:errorcluster, "refnum"=w250:T10)  [unwired: 8 in, 1 out]
        n189 = call-poly <vilib>:"Write Key.vi"("section"="CODMn参数" ("key"), "error in (no error)"=w251, "value"=w244, "key"="跨度液浓度", "refnum"=w250) -> ("error out"=w253:errorcluster, "refnum out"=w252:T10)  [unwired: 4 in, 1 out]
        n190 = call <vilib>:"Close Config Data.vi"("error in (no error)"=w253, "refnum"=w252) -> ()  [unwired: 8 in, 2 out]
      }
      event "泵滴定数1": Mouse Down {
        n191 = event-data() -> ()  [unwired: 1 in, 8 out]
        n192 = local read "泵滴定数1"() -> (w255:dbl)
        n193 = call "数字键盘.vi"("OldNumber"=w255) -> ("NewNumber"=w254:sgl)
        n194 = property on="泵滴定数1" class="DigNum (严格)"("Val(Sgnl)"=w254) -> ()  [unwired: 2 in, 2 out]
      }
      event "泵滴定数2": Mouse Down {
        n195 = event-data() -> ()  [unwired: 1 in, 8 out]
        n196 = local read "泵滴定数2"() -> (w257:dbl)
        n197 = call "数字键盘.vi"("OldNumber"=w257) -> ("NewNumber"=w256:sgl)
        n198 = property on="泵滴定数2" class="DigNum (严格)"("Val(Sgnl)"=w256) -> ()  [unwired: 2 in, 2 out]
      }
      event "泵滴定数3": Mouse Down {
        n199 = event-data() -> ()  [unwired: 1 in, 8 out]
        n200 = local read "泵滴定数3"() -> (w259:dbl)
        n201 = call "数字键盘.vi"("OldNumber"=w259) -> ("NewNumber"=w258:sgl)
        n202 = property on="泵滴定数3" class="DigNum (严格)"("Val(Sgnl)"=w258) -> ()  [unwired: 2 in, 2 out]
      }
      event "泵滴定数4": Mouse Down {
        n203 = event-data() -> ()  [unwired: 1 in, 8 out]
        n204 = local read "泵滴定数4"() -> (w261:dbl)
        n205 = call "数字键盘.vi"("OldNumber"=w261) -> ("NewNumber"=w260:sgl)
        n206 = property on="泵滴定数4" class="DigNum (严格)"("Val(Sgnl)"=w260) -> ()  [unwired: 2 in, 2 out]
      }
      event "泵滴定数5": Mouse Down {
        n207 = event-data() -> ()  [unwired: 1 in, 8 out]
        n208 = local read "泵滴定数5"() -> (w263:dbl)
        n209 = call "数字键盘.vi"("OldNumber"=w263) -> ("NewNumber"=w262:sgl)
        n210 = property on="泵滴定数5" class="DigNum (严格)"("Val(Sgnl)"=w262) -> ()  [unwired: 2 in, 2 out]
      }
      event "低切高阈值", "高切低阈值": Mouse Down {
        n211 = event-data() -> ("CtlRef"=w267:refnum<vi>)  [unwired: 1 in, 7 out]
        n212 = property class="DigNum (严格)"(reference=w267) -> (reference out=w266:refnum<vi>, "Value"=w265:dbl)  [unwired: 1 in, 1 out]
        n213 = call "数字键盘.vi"("OldNumber"=w265) -> ("NewNumber"=w264:sgl)
        n214 = property class="DigNum (严格)"(reference=w266, "Val(Sgnl)"=w264) -> ()  [unwired: 1 in, 2 out]
      }
    }
  }
  n215 = call <vilib>:"Application Directory.vi"() -> ("Application Directory"=w4:path)
  n216 = Build Path(base path=w4, name or relative path="data\\sys.ini" ("名称或相对路径")) -> (appended path=w6:path)
  n217 = call <vilib>:"Open Config Data.vi"("configuration file path"=w6) -> ("error out"=w10:errorcluster, "refnum"=w7:T10)  [unwired: 8 in, 1 out]
  n218 = vi-ref "斯坦道CODMn.lvlib:CODMn断电保存全局变量.vi"() -> (w8:refnum<vi>)
  n219 = call <userlib>:"Read Panel from INI__ogtk.vi"("error in (no error)"=w10, "VI ref"=w8, "refnum"=w7) -> ("error out"=w11:errorcluster, "refnum out"=w9:T10)  [unwired: 7 in]
  n220 = global write "COD浓度全局变量.vi" "VISA resource name"("VISA resource name") -> ()
  n221 = call <vilib>:"Close Config Data.vi"("error in (no error)"=w11, "refnum"=w9) -> ("error out"=w12:errorcluster, "file path"=w13:path)  [unwired: 8 in]
  n222 = Open/Create/Replace File(file path (use dialog)=w13, error in=w12) -> (error out=w3:errorcluster)  [unwired: 4 in, 2 out]
  n223 = call <vilib>:"Open Serial Session.vi"("Mode (RTU)"=enum16{"RTU", "ASCII"}."RTU", "Slave ID"="Slave ID", "Serial Config"="Serial Config", "VISA Resource"="VISA resource name") -> ("Error out"=w1:errorcluster, "MB_Serial session"=w2:refnum<class "MB_Master_Serial.lvclass">)  [unwired: 6 in]
  n224 = global write "COD浓度全局变量.vi" "MB_Serial session"(w2) -> ()
  n225 = global write "COD浓度全局变量.vi" "Error in"(w1) -> ()
  n226 = Obtain Queue(max queue size (-1, unlimited)=-1 ("队列最大值（-1，无限）"), name (unnamed)="读取写入DATABASE" ("名称（未命名）"), element data type=T5 {"starting address"=4224, "number of holding registers"=16}) -> (queue out=w22:refnum<queue>, error out=w21:errorcluster)  [unwired: 2 in, 1 out]
  n227 = Obtain Queue(max queue size (-1, unlimited)=-1 ("队列最大值（-1，无限）"), name (unnamed)="读取参数" ("名称（未命名）"), element data type=T5 {"starting address"=4224, "number of holding registers"=16}) -> (queue out=w15:refnum<queue>, error out=w14:errorcluster)  [unwired: 2 in, 1 out]
  n228 = Obtain Queue(max queue size (-1, unlimited)=-1 ("队列最大值（-1，无限）"), name (unnamed)="写入" ("名称（未命名）"), element data type=cluster{"starting address":u16, "values":u16[]} {"starting address"=4272, "values"=[]}) -> (queue out=w18:refnum<queue>, error out=w20:errorcluster)  [unwired: 2 in, 1 out]
  n229 = Obtain Queue(max queue size (-1, unlimited)=-1 ("队列最大值（-1，无限）"), name (unnamed)="读取" ("名称（未命名）"), element data type=T5 {"starting address"=4224, "number of holding registers"=16}) -> (queue out=w32:refnum<queue>, error out=w31:errorcluster)  [unwired: 2 in, 1 out]
  n230 = while {
    tunnel: w32 -> [w275]
    tunnel: w31 -> [w274]
    tunnel: w18 -> [w273]
    tunnel: w15 -> [w272]
    tunnel: w14 -> [w271]
    tunnel: w2 -> [w269]
    tunnel: w1 -> [w268]
    tunnel: w3 -> [_]
    stop <- FALSE stop-if-true
    n231 = event shown="[13] \"时间校准\": 值改变" {
      selector: _ -> [_ _ _ _ _ _ _ _ _ _ _ _ _ _ _ _ _ _ _ _ _ _ _ _]
      dyn-events: _ -> [_ _ _ _ _ _ _ _ _ _ _ _ _ _ _ _ _ _ _ _ _ _ _ _]
      timeout: _ -> [_ _ _ _ _ _ _ _ _ _ _ _ _ _ _ _ _ _ _ _ _ _ _ _]
      tunnel: w275 -> [_ _ _ _ _ _ _ _ _ _ _ _ _ _ _ _ _ _ _ _ _ _ _ _]
      tunnel: w274 -> [_ _ _ _ _ _ _ _ _ _ _ _ _ _ _ _ _ _ _ _ _ _ _ _]
      tunnel: w273 -> [w283 w316 w353 _ _ w395 _ _ _ _ _ _ _ w755 w769 _ w791 _ _ _ _ w978 _ _]
      tunnel: w272 -> [_ _ _ _ w386 _ _ _ _ _ _ _ _ _ _ _ _ _ _ _ w970 _ _ _]
      tunnel: w271 -> [_ _ _ _ w385 _ _ _ _ _ _ _ _ _ _ _ _ _ _ _ w969 _ _ _]
      tunnel: w269 -> [_ _ _ w359 _ _ _ _ _ _ _ _ w754 _ _ _ _ _ _ _ _ _ _ _]
      tunnel: w268 -> [_ _ _ w358 _ _ _ _ _ _ _ _ w753 _ _ _ _ _ _ _ _ _ _ _]
      event "单步启动": Mouse Down {
        n232 = event-data() -> ()  [unwired: 1 in, 8 out]
        n233 = call "单步启动选择对话框.vi"() -> ("启动选择2"=w276:u16)  [unwired: 10 in, 1 out]
        n234 = case shown="3" w276 {
          tunnel: [u16 4610 ("address") u16 4610 ("address") u16 4610 ("address") u16 4610 ("address") u16 4610 ("address") u16 4610 ("address") u16 4610 ("address") u16 4610 ("address") u16 4610 ("address") u16 4610 ("address") u16 4610 ("address") u16 4610 ("address") u16 4610 ("address")] -> w282
          tunnel: [u16 1 ("address") u16 2 ("address") u16 3 ("address") u16 4 ("address") u16 5 ("address") u16 6 ("address") u16 7 ("address") u16 8 ("address") u16 9 ("holding register value") u16 10 ("holding register value") u16 11 ("holding register value") u16 12 ("address") u16 0 ("address")] -> w279
          frame 0 {
          }
          frame 1 {
          }
          frame 2 {
          }
          frame 3 {
          }
          frame 4 {
          }
          frame 5 {
          }
          frame 6 {
          }
          frame 7 {
          }
          frame 8 {
          }
          frame 9 {
          }
          frame 10 {
          }
          frame 11 {
          }
          frame 12, Default {
          }
        }
        n235 = local write "枚举"(enum16{"读取数据", "写入数据", "读取写入DATABASE", "读取参数"}."写入数据" ("枚举")) -> ()
        n236 = Insert Into Array(array=u16[] [] ("values"), index=0 ("索引"), new element=w279) -> (w278:u16[])
        n237 = Bundle By Name(cluster=cluster{"starting address":u16, "values":u16[]} {"starting address"=0, "values"=[]}, "starting address"=w282, "values"=w278) -> (w284:cluster{"starting address":u16, "values":u16[]})
        n238 = Enqueue Element(queue=w283, element=w284) -> ()  [unwired: 2 in, 3 out]
      }
      event "启动": Mouse Down {
        n239 = event-data() -> ()  [unwired: 1 in, 8 out]
        n240 = flat-sequence {
          tunnel: w316 -> [w319]
          tunnel: [w319] -> w315
          tunnel: [w318] -> w312
          tunnel: w315 -> [w322]
          tunnel: [w322] -> w314
          tunnel: [w320] -> w313
          tunnel: w312 -> [w320]
          tunnel: w314 -> [w324]
          tunnel: w313 -> [w323]
          frame #0 {
            n241 = call "启动测量模式选择对话框.vi"() -> ("启动选择 2"=w318:u16)  [unwired: 11 in]
            "启动选择 2" <- w318
          }
          frame #1 {
            n242 = property on="启动选择 2" class="Ring (严格)"() -> ("RingText.Text"=w321:string)  [unwired: 2 in, 2 out]
            n243 = global write "COD测量模式全局.vi" "测量模式"(w321) -> ()
          }
          frame #2 {
            n244 = case shown="9, 默认" w323 {
              tunnel: [u16 4608 ("address") u16 4608 ("address") u16 4608 ("address") u16 4608 ("address") u16 4608 ("address") u16 4608 ("address") u16 4608 ("address") u16 4608 ("address") u16 4608 ("address") u16 4608 ("address")] -> w325
              tunnel: [u16 1 ("address") u16 2 ("address") u16 3 ("address") u16 4 ("address") u16 5 ("address") u16 7 ("address") u16 6 ("address") u16 8 ("address") u16 9 ("address") u16 0 ("address")] -> w326
              frame 0 {
              }
              frame 1 {
              }
              frame 2 {
              }
              frame 3 {
              }
              frame 4 {
              }
              frame 5 {
              }
              frame 6 {
              }
              frame 7 {
              }
              frame 8 {
              }
              frame 9, Default {
              }
            }
            n245 = Insert Into Array(array=u16[] [] ("values"), index=0 ("索引"), new element=w326) -> (w331:u16[])
            n246 = Bundle By Name(cluster=cluster{"starting address":u16, "values":u16[]} {"starting address"=0, "values"=[]}, "starting address"=w325, "values"=w331) -> (w328:cluster{"starting address":u16, "values":u16[]})
            n247 = Enqueue Element(queue=w324, element=w328) -> ()  [unwired: 2 in, 3 out]
          }
        }
        n248 = local write "枚举"(enum16{"读取数据", "写入数据", "读取写入DATABASE", "读取参数"}."写入数据" ("枚举")) -> ()
      }
      event "停止": Value Change {
        n249 = event-data() -> ()  [unwired: 1 in, 6 out]
        n250 = local write "枚举"(enum16{"读取数据", "写入数据", "读取写入DATABASE", "读取参数"}."写入数据" ("枚举")) -> ()
        n251 = Bundle By Name(cluster=cluster{"starting address":u16, "values":u16[]} {"starting address"=0, "values"=[]}, "starting address"=u16 4608, "values"=u16[] [11]) -> (w355:cluster{"starting address":u16, "values":u16[]})
        n252 = Enqueue Element(queue=w353, element=w355) -> ()  [unwired: 2 in, 3 out]
      }
      event "手动控制": Value Change {
        n253 = event-data() -> ()  [unwired: 1 in, 6 out]
        n254 = call "数字密码键盘.vi"() -> ("NewNumber"=w360:sgl)  [unwired: 1 in]
        n255 = Equal?(x=w360, y=8.0) -> (x = y?=w361:bool)
        n256 = case shown="真" w361 {
          tunnel: w359 -> [_ w365]
          tunnel: w358 -> [_ w364]
          frame False {
            n257 = call "窗口弹出对话框(子VI).vi"("消息"="密码错误") -> ()  [unwired: 10 in, 1 out]
          }
          frame True {
            n258 = call "CODMn手动控制框.vi"("Error in"=w364, "MB_Serial session"=w365) -> ()  [unwired: 10 in]
          }
        }
      }
      event "参数配置": Value Change {
        w372 = "CODMn是否切换量程" ("key")
        n259 = event-data() -> ()  [unwired: 1 in, 6 out]
        n260 = property on="窗格" class="Pane"("Origin"=T9 {"Horizontal"=0, "Vertical"=650} ("原点")) -> ()  [unwired: 2 in, 2 out]
        n261 = Bundle By Name(cluster=T5 {"starting address"=0, "number of holding registers"=0}, "starting address"=u16 4240, "number of holding registers"=u16 16) -> (w393:T5)
        n262 = local write "读取KB值"(FALSE ("读取KB值")) -> ()
        n263 = local write "枚举"(enum16{"读取数据", "写入数据", "读取写入DATABASE", "读取参数"}."读取参数" ("枚举")) -> ()
        n264 = Flush Queue(queue=w386, error in (no error)=w385) -> (queue out=w389:refnum<queue>, error out=w388:errorcluster)  [unwired: 1 out]
        n265 = Enqueue Element(queue=w389, element=w393, error in (no error)=w388) -> ()  [unwired: 1 in, 3 out]
        n266 = call <vilib>:"Application Directory.vi"() -> ("Application Directory"=w381:path)
        n267 = Build Path(base path=w381, name or relative path="data\\Set.ini" ("名称或相对路径")) -> (appended path=w379:path)
        n268 = call <vilib>:"Open Config Data.vi"("configuration file path"=w379) -> ("error out"=w382:errorcluster, "refnum"=w383:T10)  [unwired: 8 in, 1 out]
        n269 = call-poly <vilib>:"Read Key.vi"("section"=w372, "error in (no error)"=w382, "key"="自动切换量程", "refnum"=w383) -> ("error out"=w375:errorcluster, "value"=w377:bool, "refnum out"=w376:T10)  [unwired: 4 in, 1 out]
        n270 = local write "自动切换量程"(w377) -> ()
        n271 = call-poly <vilib>:"Read Key.vi"("section"=w372, "error in (no error)"=w375, "key"="低切高阈值", "refnum"=w376) -> ("error out"=w373:errorcluster, "value"=w367:dbl, "refnum out"=w374:T10)  [unwired: 4 in, 1 out]
        n272 = local write "低切高阈值"(w367) -> ()
        n273 = call-poly <vilib>:"Read Key.vi"("section"=w372, "error in (no error)"=w373, "key"="高切低阈值", "refnum"=w374) -> ("error out"=w370:errorcluster, "value"=w366:dbl, "refnum out"=w371:T10)  [unwired: 4 in, 1 out]
        n274 = local write "高切低阈值"(w366) -> ()
        n275 = call <vilib>:"Close Config Data.vi"("error in (no error)"=w370, "refnum"=w371) -> ()  [unwired: 8 in, 2 out]
      }
      event "保存": Mouse Down {
        n276 = event-data() -> ()  [unwired: 1 in, 8 out]
        n277 = call <vilib>:"Application Directory.vi"() -> ("Application Directory"=w421:path)
        n278 = Build Path(base path=w421, name or relative path="data\\Set.ini" ("名称或相对路径")) -> (appended path=w423:path)
        n279 = local write "枚举"(enum16{"读取数据", "写入数据", "读取写入DATABASE", "读取参数"}."写入数据" ("枚举")) -> ()
        n280 = local read "跨度液浓度"() -> (w418:dbl)
        n281 = call <vilib>:"Open Config Data.vi"("configuration file path"=w423) -> ("error out"=w425:errorcluster, "refnum"=w424:T10)  [unwired: 8 in, 1 out]
        n282 = call-poly <vilib>:"Write Key.vi"("section"="CODMn参数" ("key"), "error in (no error)"=w425, "value"=w418, "key"="跨度液浓度", "refnum"=w424) -> ("error out"=w427:errorcluster, "refnum out"=w426:T10)  [unwired: 4 in, 1 out]
        n283 = call <vilib>:"Close Config Data.vi"("error in (no error)"=w427, "refnum"=w426) -> ()  [unwired: 8 in, 2 out]
        n284 = local write "水样"("水样") -> ()
        n285 = local write "标液"("标液") -> ()
        n286 = local write "硫酸"("硫酸") -> ()
        n287 = local write "恒温时间"("恒温时间") -> ()
        n288 = local write "修正系数"("修正系数") -> ()
        n289 = local write "加标回收"("加标回收") -> ()
        n290 = local write "高锰酸钾"("高锰酸钾") -> ()
        n291 = local write "基本量程"("基本量程") -> ()
        n292 = local write "标样浓度 2"("标样浓度 2") -> ()
        n293 = local write "零点泵计量数 2"("零点泵计量数 2") -> ()
        n294 = local write "标度泵计量数 2"("标度泵计量数 2") -> ()
        n295 = local write "温度 2"("温度 2") -> ()
        n296 = local write "蒸馏水"("蒸馏水") -> ()
        n297 = local write "草酸钠"("草酸钠") -> ()
        n298 = local write "质控样"("质控样") -> ()
        n299 = Build Array("温度 2", "恒温时间", "浓度", "修正系数", "基本量程", "水样", "蒸馏水", "标液", "质控样", "加标回收", "高锰酸钾", "草酸钠", "硫酸", "零点泵计量数 2", "标度泵计量数 2", "标样浓度 2") -> (w410:dbl[])
        n300 = Bundle By Name(cluster=cluster{"starting address":u16, "values":u16[]} {"starting address"=4272, "values"=[]}, "starting address"=u16 4272, "values"=w410) -> (w412:cluster{"starting address":u16, "values":u16[]})
        n301 = Enqueue Element(queue=w395, element=w412, timeout in ms (-1)=1000 ("超时毫秒(-1)")) -> ()  [unwired: 1 in, 3 out]
      }
      event "校准配置": Value Change {
        n302 = event-data() -> ()  [unwired: 1 in, 6 out]
        n303 = property on="窗格" class="Pane"("Origin"=T9 {"Horizontal"=0, "Vertical"=1300} ("原点")) -> ()  [unwired: 2 in, 2 out]
        n304 = call <vilib>:"Application Directory.vi"() -> ("Application Directory"=w478:path)
        n305 = Build Path(base path=w478, name or relative path="data\\Set.ini" ("名称或相对路径")) -> (appended path=w476:path)
        n306 = call <vilib>:"Open Config Data.vi"("configuration file path"=w476) -> ("error out"=w446:errorcluster, "refnum"=w447:T10)  [unwired: 8 in, 1 out]
        n307 = call-poly <vilib>:"Read Key.vi"("section"="CODMn模型选择" ("key"), "error in (no error)"=w446, "key"="线性和多项式", "refnum"=w447) -> ("error out"=w442:errorcluster, "value"=w445:i32, "refnum out"=w443:T10)  [unwired: 4 in, 1 out]
        n308 = local write "模型"(w445) -> ()
        n309 = call-poly <vilib>:"Read Key.vi"("section"="标线选择", "error in (no error)"=w442, "key"="选用水样", "refnum"=w443) -> ("error out"=w440:errorcluster, "value"=w444:i32, "refnum out"=w441:T10)  [unwired: 4 in, 1 out]
        n310 = local write "选用水样"(w444) -> ()
        n311 = local read "量程选择"() -> (w453:enum16{"低量程", "高量程", "0-2量程"})
        n312 = case shown="0, 默认" w444 {
          tunnel: ["葡萄糖标线" ("section") "草酸钠标线" ("section")] -> w452
          frame 0, Default {
          }
          frame 1 {
          }
        }
        n313 = case shown="\"0-2量程\"" w453 {
          tunnel: ["低量程" "高量程" "0-2量程"] -> w451
          frame "低量程", Default {
          }
          frame "高量程" {
          }
          frame "0-2量程" {
          }
        }
        n314 = Concatenate Strings(w452, w451) -> (w450:string)
        n315 = call-poly <vilib>:"Read Key.vi"("section"=w450, "error in (no error)"=w440, "key"="浓度1", "refnum"=w441) -> ("error out"=w482:errorcluster, "value"=w480:dbl, "refnum out"=w481:T10)  [unwired: 4 in, 1 out]
        n316 = local write "浓度1"(w480) -> ()
        n317 = call-poly <vilib>:"Read Key.vi"("section"=w450, "error in (no error)"=w482, "key"="浓度2", "refnum"=w481) -> ("error out"=w496:errorcluster, "value"=w483:dbl, "refnum out"=w495:T10)  [unwired: 4 in, 1 out]
        n318 = local write "浓度2"(w483) -> ()
        n319 = call-poly <vilib>:"Read Key.vi"("section"=w450, "error in (no error)"=w496, "key"="浓度3", "refnum"=w495) -> ("error out"=w497:errorcluster, "value"=w485:dbl, "refnum out"=w494:T10)  [unwired: 4 in, 1 out]
        n320 = local write "浓度3"(w485) -> ()
        n321 = call-poly <vilib>:"Read Key.vi"("section"=w450, "error in (no error)"=w497, "key"="泵滴定数1", "refnum"=w494) -> ("error out"=w498:errorcluster, "value"=w487:dbl, "refnum out"=w493:T10)  [unwired: 4 in, 1 out]
        n322 = local write "泵滴定数1"(w487) -> ()
        n323 = call-poly <vilib>:"Read Key.vi"("section"=w450, "error in (no error)"=w498, "key"="泵滴定数2", "refnum"=w493) -> ("error out"=w492:errorcluster, "value"=w490:dbl, "refnum out"=w499:T10)  [unwired: 4 in, 1 out]
        n324 = local write "泵滴定数2"(w490) -> ()
        n325 = call-poly <vilib>:"Read Key.vi"("section"=w450, "error in (no error)"=w492, "key"="泵滴定数3", "refnum"=w499) -> ("error out"=w504:errorcluster, "value"=w503:dbl, "refnum out"=w500:T10)  [unwired: 4 in, 1 out]
        n326 = local write "泵滴定数3"(w503) -> ()
        n327 = call-poly <vilib>:"Read Key.vi"("section"=w450, "error in (no error)"=w504, "key"="浓度4", "refnum"=w500) -> ("error out"=w505:errorcluster, "value"=w433:dbl, "refnum out"=w501:T10)  [unwired: 4 in, 1 out]
        n328 = local write "浓度4"(w433) -> ()
        n329 = call-poly <vilib>:"Read Key.vi"("section"=w450, "error in (no error)"=w505, "key"="浓度5", "refnum"=w501) -> ("error out"=w438:errorcluster, "value"=w432:dbl, "refnum out"=w439:T10)  [unwired: 4 in, 1 out]
        n330 = local write "浓度5"(w432) -> ()
        n331 = call-poly <vilib>:"Read Key.vi"("section"=w450, "error in (no error)"=w438, "key"="泵滴定数4", "refnum"=w439) -> ("error out"=w506:errorcluster, "value"=w431:dbl, "refnum out"=w502:T10)  [unwired: 4 in, 1 out]
        n332 = local write "泵滴定数4"(w431) -> ()
        n333 = call-poly <vilib>:"Read Key.vi"("section"=w450, "error in (no error)"=w506, "key"="泵滴定数5", "refnum"=w502) -> ("error out"=w436:errorcluster, "value"=w430:dbl, "refnum out"=w437:T10)  [unwired: 4 in, 1 out]
        n334 = local write "泵滴定数5"(w430) -> ()
        n335 = call-poly <vilib>:"Read Key.vi"("section"=w450, "error in (no error)"=w436, "key"="当前选用的校准", "refnum"=w437) -> ("error out"=w472:errorcluster, "value"=w474:i32, "refnum out"=w473:T10)  [unwired: 4 in, 1 out]
        n336 = local write "当前校准"(w474) -> ()
        n337 = call-poly <vilib>:"Read Key.vi"("section"=w450, "error in (no error)"=w472, "key"="启用1", "refnum"=w473) -> ("error out"=w469:errorcluster, "value"=w458:bool, "refnum out"=w470:T10)  [unwired: 4 in, 1 out]
        n338 = local write "启用1"(w458) -> ()
        n339 = call-poly <vilib>:"Read Key.vi"("section"=w450, "error in (no error)"=w469, "key"="启用2", "refnum"=w470) -> ("error out"=w467:errorcluster, "value"=w457:bool, "refnum out"=w468:T10)  [unwired: 4 in, 1 out]
        n340 = local write "启用2"(w457) -> ()
        n341 = call-poly <vilib>:"Read Key.vi"("section"=w450, "error in (no error)"=w467, "key"="启用3", "refnum"=w468) -> ("error out"=w465:errorcluster, "value"=w456:bool, "refnum out"=w466:T10)  [unwired: 4 in, 1 out]
        n342 = local write "启用3"(w456) -> ()
        n343 = call-poly <vilib>:"Read Key.vi"("section"=w450, "error in (no error)"=w465, "key"="启用4", "refnum"=w466) -> ("error out"=w463:errorcluster, "value"=w429:bool, "refnum out"=w464:T10)  [unwired: 4 in, 1 out]
        n344 = local write "启用4"(w429) -> ()
        n345 = call-poly <vilib>:"Read Key.vi"("section"=w450, "error in (no error)"=w463, "key"="启用5", "refnum"=w464) -> ("error out"=w434:errorcluster, "value"=w428:bool, "refnum out"=w435:T10)  [unwired: 4 in, 1 out]
        n346 = local write "启用5"(w428) -> ()
        n347 = call <vilib>:"Close Config Data.vi"("error in (no error)"=w434, "refnum"=w435) -> ()  [unwired: 8 in, 2 out]
      }
      event "选用水样": Value Change {
        (unwired) "浓度6" ("key")
        n348 = event-data() -> ()  [unwired: 1 in, 6 out]
        n349 = property on="窗格" class="Pane"("Origin"=T9 {"Horizontal"=0, "Vertical"=1300} ("原点")) -> ()  [unwired: 2 in, 2 out]
        n350 = local read "量程选择"() -> (w530:enum16{"低量程", "高量程", "0-2量程"})
        n351 = case shown="\"0-2量程\"" w530 {
          tunnel: ["低量程" "高量程" "0-2量程"] -> w531
          frame "低量程", Default {
          }
          frame "高量程" {
          }
          frame "0-2量程" {
          }
        }
        n352 = case shown="\"葡萄糖\", 默认" "选用水样" {
          tunnel: ["葡萄糖标线" ("section") "草酸钠标线" ("section")] -> w532
          frame "葡萄糖", Default {
          }
          frame "草酸钠" {
          }
        }
        n353 = call <vilib>:"Application Directory.vi"() -> ("Application Directory"=w556:path)
        n354 = Build Path(base path=w556, name or relative path="data\\Set.ini" ("名称或相对路径")) -> (appended path=w554:path)
        n355 = call <vilib>:"Open Config Data.vi"("configuration file path"=w554) -> ("error out"=w557:errorcluster, "refnum"=w558:T10)  [unwired: 8 in, 1 out]
        n356 = Concatenate Strings(w532, w531) -> (w529:string)
        n357 = call-poly <vilib>:"Read Key.vi"("section"=w529, "error in (no error)"=w557, "key"="浓度1", "refnum"=w558) -> ("error out"=w562:errorcluster, "value"=w560:dbl, "refnum out"=w561:T10)  [unwired: 4 in, 1 out]
        n358 = local write "浓度1"(w560) -> ()
        n359 = call-poly <vilib>:"Read Key.vi"("section"=w529, "error in (no error)"=w562, "key"="浓度2", "refnum"=w561) -> ("error out"=w576:errorcluster, "value"=w563:dbl, "refnum out"=w575:T10)  [unwired: 4 in, 1 out]
        n360 = local write "浓度2"(w563) -> ()
        n361 = call-poly <vilib>:"Read Key.vi"("section"=w529, "error in (no error)"=w576, "key"="浓度3", "refnum"=w575) -> ("error out"=w577:errorcluster, "value"=w565:dbl, "refnum out"=w574:T10)  [unwired: 4 in, 1 out]
        n362 = local write "浓度3"(w565) -> ()
        n363 = call-poly <vilib>:"Read Key.vi"("section"=w529, "error in (no error)"=w577, "key"="泵滴定数1", "refnum"=w574) -> ("error out"=w578:errorcluster, "value"=w567:dbl, "refnum out"=w573:T10)  [unwired: 4 in, 1 out]
        n364 = local write "泵滴定数1"(w567) -> ()
        n365 = call-poly <vilib>:"Read Key.vi"("section"=w529, "error in (no error)"=w578, "key"="泵滴定数2", "refnum"=w573) -> ("error out"=w572:errorcluster, "value"=w570:dbl, "refnum out"=w579:T10)  [unwired: 4 in, 1 out]
        n366 = local write "泵滴定数2"(w570) -> ()
        n367 = call-poly <vilib>:"Read Key.vi"("section"=w529, "error in (no error)"=w572, "key"="泵滴定数3", "refnum"=w579) -> ("error out"=w584:errorcluster, "value"=w583:dbl, "refnum out"=w580:T10)  [unwired: 4 in, 1 out]
        n368 = local write "泵滴定数3"(w583) -> ()
        n369 = call-poly <vilib>:"Read Key.vi"("section"=w529, "error in (no error)"=w584, "key"="浓度4", "refnum"=w580) -> ("error out"=w585:errorcluster, "value"=w524:dbl, "refnum out"=w581:T10)  [unwired: 4 in, 1 out]
        n370 = local write "浓度4"(w524) -> ()
        n371 = call-poly <vilib>:"Read Key.vi"("section"=w529, "error in (no error)"=w585, "key"="浓度5", "refnum"=w581) -> ("error out"=w527:errorcluster, "value"=w523:dbl, "refnum out"=w528:T10)  [unwired: 4 in, 1 out]
        n372 = local write "浓度5"(w523) -> ()
        n373 = call-poly <vilib>:"Read Key.vi"("section"=w529, "error in (no error)"=w527, "key"="泵滴定数4", "refnum"=w528) -> ("error out"=w586:errorcluster, "value"=w522:dbl, "refnum out"=w582:T10)  [unwired: 4 in, 1 out]
        n374 = local write "泵滴定数4"(w522) -> ()
        n375 = call-poly <vilib>:"Read Key.vi"("section"=w529, "error in (no error)"=w586, "key"="泵滴定数5", "refnum"=w582) -> ("error out"=w525:errorcluster, "value"=w521:dbl, "refnum out"=w526:T10)  [unwired: 4 in, 1 out]
        n376 = local write "泵滴定数5"(w521) -> ()
        n377 = call-poly <vilib>:"Read Key.vi"("section"=w529, "error in (no error)"=w525, "key"="当前选用的校准", "refnum"=w526) -> ("error out"=w550:errorcluster, "value"=w552:i32, "refnum out"=w551:T10)  [unwired: 4 in, 1 out]
        n378 = local write "当前校准"(w552) -> ()
        n379 = call-poly <vilib>:"Read Key.vi"("section"=w529, "error in (no error)"=w550, "key"="启用1", "refnum"=w551) -> ("error out"=w547:errorcluster, "value"=w536:bool, "refnum out"=w548:T10)  [unwired: 4 in, 1 out]
        n380 = local write "启用1"(w536) -> ()
        n381 = call-poly <vilib>:"Read Key.vi"("section"=w529, "error in (no error)"=w547, "key"="启用2", "refnum"=w548) -> ("error out"=w545:errorcluster, "value"=w535:bool, "refnum out"=w546:T10)  [unwired: 4 in, 1 out]
        n382 = local write "启用2"(w535) -> ()
        n383 = call-poly <vilib>:"Read Key.vi"("section"=w529, "error in (no error)"=w545, "key"="启用3", "refnum"=w546) -> ("error out"=w543:errorcluster, "value"=w534:bool, "refnum out"=w544:T10)  [unwired: 4 in, 1 out]
        n384 = local write "启用3"(w534) -> ()
        n385 = call-poly <vilib>:"Read Key.vi"("section"=w529, "error in (no error)"=w543, "key"="启用4", "refnum"=w544) -> ("error out"=w541:errorcluster, "value"=w518:bool, "refnum out"=w542:T10)  [unwired: 4 in, 1 out]
        n386 = local write "启用4"(w518) -> ()
        n387 = call-poly <vilib>:"Read Key.vi"("section"=w529, "error in (no error)"=w541, "key"="启用5", "refnum"=w542) -> ("error out"=w519:errorcluster, "value"=w517:bool, "refnum out"=w520:T10)  [unwired: 4 in, 1 out]
        n388 = local write "启用5"(w517) -> ()
        n389 = call <vilib>:"Close Config Data.vi"("error in (no error)"=w519, "refnum"=w520) -> ()  [unwired: 8 in, 2 out]
      }
      event "量程选择": Value Change {
        n390 = event-data() -> ()  [unwired: 1 in, 6 out]
        n391 = property on="窗格" class="Pane"("Origin"=T9 {"Horizontal"=0, "Vertical"=1300} ("原点")) -> ()  [unwired: 2 in, 2 out]
        n392 = local read "选用水样"() -> (w613:enum16{"葡萄糖", "草酸钠"})
        n393 = case shown="\"葡萄糖\", 默认" w613 {
          tunnel: ["葡萄糖标线" ("section") "草酸钠标线" ("section")] -> w612
          frame "葡萄糖", Default {
          }
          frame "草酸钠" {
          }
        }
        n394 = case shown="\"0-2量程\"" "量程选择" {
          tunnel: ["低量程" "高量程" "0-2量程"] -> w609
          frame "低量程", Default {
          }
          frame "高量程" {
          }
          frame "0-2量程" {
          }
        }
        n395 = call <vilib>:"Application Directory.vi"() -> ("Application Directory"=w636:path)
        n396 = Build Path(base path=w636, name or relative path="data\\Set.ini" ("名称或相对路径")) -> (appended path=w634:path)
        n397 = call <vilib>:"Open Config Data.vi"("configuration file path"=w634) -> ("error out"=w637:errorcluster, "refnum"=w638:T10)  [unwired: 8 in, 1 out]
        n398 = Concatenate Strings(w612, w609) -> (w611:string)
        n399 = call-poly <vilib>:"Read Key.vi"("section"=w611, "error in (no error)"=w637, "key"="浓度1", "refnum"=w638) -> ("error out"=w642:errorcluster, "value"=w640:dbl, "refnum out"=w641:T10)  [unwired: 4 in, 1 out]
        n400 = local write "浓度1"(w640) -> ()
        n401 = call-poly <vilib>:"Read Key.vi"("section"=w611, "error in (no error)"=w642, "key"="浓度2", "refnum"=w641) -> ("error out"=w656:errorcluster, "value"=w643:dbl, "refnum out"=w655:T10)  [unwired: 4 in, 1 out]
        n402 = local write "浓度2"(w643) -> ()
        n403 = call-poly <vilib>:"Read Key.vi"("section"=w611, "error in (no error)"=w656, "key"="浓度3", "refnum"=w655) -> ("error out"=w657:errorcluster, "value"=w645:dbl, "refnum out"=w654:T10)  [unwired: 4 in, 1 out]
        n404 = local write "浓度3"(w645) -> ()
        n405 = call-poly <vilib>:"Read Key.vi"("section"=w611, "error in (no error)"=w657, "key"="泵滴定数1", "refnum"=w654) -> ("error out"=w658:errorcluster, "value"=w647:dbl, "refnum out"=w653:T10)  [unwired: 4 in, 1 out]
        n406 = local write "泵滴定数1"(w647) -> ()
        n407 = call-poly <vilib>:"Read Key.vi"("section"=w611, "error in (no error)"=w658, "key"="泵滴定数2", "refnum"=w653) -> ("error out"=w652:errorcluster, "value"=w650:dbl, "refnum out"=w659:T10)  [unwired: 4 in, 1 out]
        n408 = local write "泵滴定数2"(w650) -> ()
        n409 = call-poly <vilib>:"Read Key.vi"("section"=w611, "error in (no error)"=w652, "key"="泵滴定数3", "refnum"=w659) -> ("error out"=w664:errorcluster, "value"=w663:dbl, "refnum out"=w660:T10)  [unwired: 4 in, 1 out]
        n410 = local write "泵滴定数3"(w663) -> ()
        n411 = call-poly <vilib>:"Read Key.vi"("section"=w611, "error in (no error)"=w664, "key"="浓度4", "refnum"=w660) -> ("error out"=w665:errorcluster, "value"=w600:dbl, "refnum out"=w661:T10)  [unwired: 4 in, 1 out]
        n412 = local write "浓度4"(w600) -> ()
        n413 = call-poly <vilib>:"Read Key.vi"("section"=w611, "error in (no error)"=w665, "key"="浓度5", "refnum"=w661) -> ("error out"=w607:errorcluster, "value"=w599:dbl, "refnum out"=w608:T10)  [unwired: 4 in, 1 out]
        n414 = local write "浓度5"(w599) -> ()
        n415 = call-poly <vilib>:"Read Key.vi"("section"=w611, "error in (no error)"=w607, "key"="泵滴定数4", "refnum"=w608) -> ("error out"=w666:errorcluster, "value"=w598:dbl, "refnum out"=w662:T10)  [unwired: 4 in, 1 out]
        n416 = local write "泵滴定数4"(w598) -> ()
        n417 = call-poly <vilib>:"Read Key.vi"("section"=w611, "error in (no error)"=w666, "key"="泵滴定数5", "refnum"=w662) -> ("error out"=w605:errorcluster, "value"=w597:dbl, "refnum out"=w606:T10)  [unwired: 4 in, 1 out]
        n418 = local write "泵滴定数5"(w597) -> ()
        n419 = call-poly <vilib>:"Read Key.vi"("section"=w611, "error in (no error)"=w605, "key"="当前选用的校准", "refnum"=w606) -> ("error out"=w630:errorcluster, "value"=w632:i32, "refnum out"=w631:T10)  [unwired: 4 in, 1 out]
        n420 = local write "当前校准"(w632) -> ()
        n421 = call-poly <vilib>:"Read Key.vi"("section"=w611, "error in (no error)"=w630, "key"="启用1", "refnum"=w631) -> ("error out"=w627:errorcluster, "value"=w616:bool, "refnum out"=w628:T10)  [unwired: 4 in, 1 out]
        n422 = local write "启用1"(w616) -> ()
        n423 = call-poly <vilib>:"Read Key.vi"("section"=w611, "error in (no error)"=w627, "key"="启用2", "refnum"=w628) -> ("error out"=w625:errorcluster, "value"=w615:bool, "refnum out"=w626:T10)  [unwired: 4 in, 1 out]
        n424 = local write "启用2"(w615) -> ()
        n425 = call-poly <vilib>:"Read Key.vi"("section"=w611, "error in (no error)"=w625, "key"="启用3", "refnum"=w626) -> ("error out"=w623:errorcluster, "value"=w614:bool, "refnum out"=w624:T10)  [unwired: 4 in, 1 out]
        n426 = local write "启用3"(w614) -> ()
        n427 = call-poly <vilib>:"Read Key.vi"("section"=w611, "error in (no error)"=w623, "key"="启用4", "refnum"=w624) -> ("error out"=w621:errorcluster, "value"=w602:bool, "refnum out"=w622:T10)  [unwired: 4 in, 1 out]
        n428 = local write "启用4"(w602) -> ()
        n429 = call-poly <vilib>:"Read Key.vi"("section"=w611, "error in (no error)"=w621, "key"="启用5", "refnum"=w622) -> ("error out"=w603:errorcluster, "value"=w601:bool, "refnum out"=w604:T10)  [unwired: 4 in, 1 out]
        n430 = local write "启用5"(w601) -> ()
        n431 = call <vilib>:"Close Config Data.vi"("error in (no error)"=w603, "refnum"=w604) -> ()  [unwired: 8 in, 2 out]
      }
      event "周期设置": Value Change {
        n432 = event-data() -> ()  [unwired: 1 in, 6 out]
        n433 = call "数字密码键盘.vi"() -> ("NewNumber"=w677:sgl)  [unwired: 1 in]
        n434 = Equal?(x=w677, y=8.0) -> (x = y?=w678:bool)
        n435 = case shown="真" w678 {
          frame False {
            n436 = call "窗口弹出对话框(子VI).vi"("消息"="密码错误") -> ()  [unwired: 10 in, 1 out]
          }
          frame True {
            n437 = call "窗口弹出对话框(子VI).vi"("消息"="登录成功") -> ("true"=w681:bool)  [unwired: 10 in]
            n438 = case shown="真" w681 {
              frame False {
              }
              frame True {
                n439 = property on="窗格" class="Pane"("Origin"=T9 {"Horizontal"=0, "Vertical"=1950} ("原点")) -> ()  [unwired: 2 in, 2 out]
              }
            }
          }
        }
      }
      event "返回": Value Change {
        (unwired) "泵滴定数6" ("key")
        w697 = "CODMn" ("section")
        n440 = event-data() -> ()  [unwired: 1 in, 6 out]
        n441 = property on="窗格" class="Pane"("Origin"=T9 {"Horizontal"=0, "Vertical"=0} ("原点")) -> ()  [unwired: 2 in, 2 out]
        n442 = call <vilib>:"Application Directory.vi"() -> ("Application Directory"=w750:path)
        n443 = Build Path(base path=w750, name or relative path="data\\Set.ini" ("名称或相对路径")) -> (appended path=w748:path)
        n444 = local write "读取KB值"(FALSE ("读取KB值")) -> ()
        n445 = call <vilib>:"Open Config Data.vi"("configuration file path"=w748) -> ("error out"=w746:errorcluster, "refnum"=w747:T10)  [unwired: 8 in, 1 out]
        n446 = local read "浓度1"() -> (w744:dbl)
        n447 = local read "浓度2"() -> (w728:dbl)
        n448 = call-poly <vilib>:"Write Key.vi"("section"=w697, "error in (no error)"=w746, "value"=w744, "key"="浓度1", "refnum"=w747) -> ("error out"=w743:errorcluster, "refnum out"=w742:T10)  [unwired: 4 in, 1 out]
        n449 = local read "浓度3"() -> (w724:dbl)
        n450 = call-poly <vilib>:"Write Key.vi"("section"=w697, "error in (no error)"=w743, "value"=w728, "key"="浓度2", "refnum"=w742) -> ("error out"=w741:errorcluster, "refnum out"=w740:T10)  [unwired: 4 in, 1 out]
        n451 = local read "泵滴定数1"() -> (w722:dbl)
        n452 = call-poly <vilib>:"Write Key.vi"("section"=w697, "error in (no error)"=w741, "value"=w724, "key"="浓度3", "refnum"=w740) -> ("error out"=w739:errorcluster, "refnum out"=w738:T10)  [unwired: 4 in, 1 out]
        n453 = call-poly <vilib>:"Write Key.vi"("section"=w697, "error in (no error)"=w739, "value"=w722, "key"="泵滴定数1", "refnum"=w738) -> ("error out"=w737:errorcluster, "refnum out"=w736:T10)  [unwired: 4 in, 1 out]
        n454 = local read "泵滴定数2"() -> (w720:dbl)
        n455 = call-poly <vilib>:"Write Key.vi"("section"=w697, "error in (no error)"=w737, "value"=w720, "key"="泵滴定数2", "refnum"=w736) -> ("error out"=w735:errorcluster, "refnum out"=w734:T10)  [unwired: 4 in, 1 out]
        n456 = local read "泵滴定数3"() -> (w718:dbl)
        n457 = local read "浓度4"() -> (w685:dbl)
        n458 = call-poly <vilib>:"Write Key.vi"("section"=w697, "error in (no error)"=w735, "value"=w718, "key"="泵滴定数3", "refnum"=w734) -> ("error out"=w733:errorcluster, "refnum out"=w732:T10)  [unwired: 4 in, 1 out]
        n459 = call-poly <vilib>:"Write Key.vi"("section"=w697, "error in (no error)"=w733, "value"=w685, "key"="浓度4", "refnum"=w732) -> ("error out"=w726:errorcluster, "refnum out"=w727:T10)  [unwired: 4 in, 1 out]
        n460 = local read "浓度5"() -> (w684:dbl)
        n461 = call-poly <vilib>:"Write Key.vi"("section"=w697, "error in (no error)"=w726, "value"=w684, "key"="浓度5", "refnum"=w727) -> ("error out"=w694:errorcluster, "refnum out"=w695:T10)  [unwired: 4 in, 1 out]
        n462 = local read "泵滴定数4"() -> (w686:dbl)
        n463 = call-poly <vilib>:"Write Key.vi"("section"=w697, "error in (no error)"=w694, "value"=w686, "key"="泵滴定数4", "refnum"=w695) -> ("error out"=w731:errorcluster, "refnum out"=w730:T10)  [unwired: 4 in, 1 out]
        n464 = local read "泵滴定数5"() -> (w687:dbl)
        n465 = call-poly <vilib>:"Write Key.vi"("section"=w697, "error in (no error)"=w731, "value"=w687, "key"="泵滴定数5", "refnum"=w730) -> ("error out"=w692:errorcluster, "refnum out"=w693:T10)  [unwired: 4 in, 1 out]
        n466 = local read "启用1"() -> (w706:bool)
        n467 = call-poly <vilib>:"Write Key.vi"("section"=w697, "error in (no error)"=w692, "value"=w706, "key"="启用1", "refnum"=w693) -> ("error out"=w702:errorcluster, "refnum out"=w705:T10)  [unwired: 4 in, 1 out]
        n468 = local read "启用2"() -> (w703:bool)
        n469 = call-poly <vilib>:"Write Key.vi"("section"=w697, "error in (no error)"=w702, "value"=w703, "key"="启用2", "refnum"=w705) -> ("error out"=w713:errorcluster, "refnum out"=w712:T10)  [unwired: 4 in, 1 out]
        n470 = local read "启用3"() -> (w701:bool)
        n471 = call-poly <vilib>:"Write Key.vi"("section"=w697, "error in (no error)"=w713, "value"=w701, "key"="启用3", "refnum"=w712) -> ("error out"=w711:errorcluster, "refnum out"=w710:T10)  [unwired: 4 in, 1 out]
        n472 = local read "启用4"() -> (w689:bool)
        n473 = call-poly <vilib>:"Write Key.vi"("section"=w697, "error in (no error)"=w711, "value"=w689, "key"="启用4", "refnum"=w710) -> ("error out"=w709:errorcluster, "refnum out"=w708:T10)  [unwired: 4 in, 1 out]
        n474 = local read "启用5"() -> (w688:bool)
        n475 = call-poly <vilib>:"Write Key.vi"("section"=w697, "error in (no error)"=w709, "value"=w688, "key"="启用5", "refnum"=w708) -> ("error out"=w690:errorcluster, "refnum out"=w691:T10)  [unwired: 4 in, 1 out]
        n476 = call <vilib>:"Close Config Data.vi"("error in (no error)"=w690, "refnum"=w691) -> ()  [unwired: 8 in, 2 out]
      }
      event "关闭", "关闭 2", "关闭 3": Value Change {
        n477 = event-data() -> ()  [unwired: 1 in, 6 out]
        n478 = property on="窗格" class="Pane"("Origin"=T9 {"Horizontal"=0, "Vertical"=0} ("原点")) -> ()  [unwired: 2 in, 2 out]
      }
      event Timeout; Application Instance Close {
        n479 = event-data() -> ()  [unwired: 1 in, 3 out]
        n480 = call-dynamic "Close Session.vi"("error in (no error)"=w753, "MB_Serial session"=w754) -> ()  [unwired: 9 in, 1 out]
      }
      event "时间校准": Value Change {
        n481 = event-data() -> ()  [unwired: 1 in, 6 out]
        n482 = flat-sequence {
          tunnel: w755 -> [w760]
          frame #0 {
            n483 = Get Date/Time In Seconds() -> (seconds since 1Jan1904=w765:timestamp)
            n484 = Build Array(w765) -> (w764:timestamp[])
            n485 = call "DateToHex.vi"("DATE"=w764) -> ("数组"=w758:u16[])  [unwired: 10 in]
            n486 = Insert Into Array(array=u16[] [1] ("values"), index=1 ("索引"), new element=w758) -> (w756:u16[])
            n487 = Bundle By Name(cluster=cluster{"starting address":u16, "values":u16[]} {"starting address"=0, "values"=[]}, "starting address"=u16 4612, "values"=w756) -> (w761:cluster{"starting address":u16, "values":u16[]})
            n488 = Enqueue Element(queue=w760, element=w761) -> ()  [unwired: 2 in, 3 out]
          }
          frame #1 {
            n489 = local write "枚举"(enum16{"读取数据", "写入数据", "读取写入DATABASE", "读取参数"}."写入数据" ("枚举")) -> ()
          }
        }
      }
      event "故障清除": Value Change {
        n490 = event-data() -> ()  [unwired: 1 in, 6 out]
        n491 = local write "枚举"(enum16{"读取数据", "写入数据", "读取写入DATABASE", "读取参数"}."写入数据" ("枚举")) -> ()
        n492 = Bundle By Name(cluster=cluster{"starting address":u16, "values":u16[]} {"starting address"=0, "values"=[]}, "starting address"=u16 4611, "values"=u16[] [1]) -> (w770:cluster{"starting address":u16, "values":u16[]})
        n493 = Enqueue Element(queue=w769, element=w770) -> ()  [unwired: 2 in, 3 out]
      }
      event "定时启动": Mouse Down {
        n494 = event-data() -> ()  [unwired: 1 in, 8 out]
        n495 = flat-sequence {
          frame #0 {
            n496 = global read "CODMn断电保存全局变量.vi" "定时控制"() -> (w773:T7)
            n497 = call "周期设置.vi"("定时控制参数输入"=w773) -> ("定时控制参数输出"=w774:T7)  [unwired: 10 in]
            n498 = global write "CODMn断电保存全局变量.vi" "定时控制"(w774) -> ()
          }
          frame #1 {
            n499 = call <vilib>:"Application Directory.vi"() -> ("Application Directory"=w788:path)
            n500 = Build Path(base path=w788, name or relative path="data\\sys.ini" ("名称或相对路径")) -> (appended path=w786:path)
            n501 = call <vilib>:"Open Config Data.vi"("configuration file path"=w786) -> ("error out"=w782:errorcluster, "refnum"=w785:T10)  [unwired: 8 in, 1 out]
            n502 = vi-ref "斯坦道CODMn.lvlib:CODMn断电保存全局变量.vi"() -> (w784:refnum<vi>)
            n503 = call <userlib>:"Write Panel to INI__ogtk.vi"("error in (no error)"=w782, "VI ref"=w784, "refnum"=w785) -> ("error out"=w781:errorcluster, "refnum out"=w783:T10)  [unwired: 7 in]
            n504 = call <vilib>:"Close Config Data.vi"("error in (no error)"=w781, "refnum"=w783) -> ("error out"=w776:errorcluster, "file path"=w775:path)  [unwired: 8 in]
            n505 = Open/Create/Replace File(file path (use dialog)=w775, error in=w776) -> (refnum out=w779:refnum<file>, error out=w780:errorcluster)  [unwired: 4 in, 1 out]
            n506 = Flush File(refnum=w779, error in=w780) -> (refnum out=w778:refnum<file>, error out=w777:errorcluster)
            n507 = Close File(refnum=w778, error in=w777) -> ()  [unwired: 2 out]
          }
        }
      }
      event "校准1", "校准2", "校准3", "校准4", "校准5": Value Change {
        n508 = event-data() -> ()  [unwired: 1 in, 6 out]
        n509 = flat-sequence {
          tunnel: w791 -> [w796]
          tunnel: [w795] -> w790
          tunnel: [w794] -> w789
          tunnel: w790 -> [w829]
          tunnel: w789 -> [w828]
          frame #0 {
            n510 = Build Array("校准1", "校准2", "校准3", "校准4", "校准5") -> (w797:bool[])
            n511 = for {
              tunnel: w797 -> [w811] mode=indexing
              tunnel: w796 -> [w807]
              tunnel: [w803] -> w795
              tunnel: [w802] -> w794
              i -> [w801]
              n512 = case shown="4" w801 {
                tunnel: ["浓度1" "浓度2" "浓度3" "浓度4" "浓度5"] -> w806
                frame 0, Default {
                }
                frame 1 {
                }
                frame 2 {
                }
                frame 3 {
                }
                frame 4 {
                }
              }
              n513 = Multiply(x=w806, y=100.0) -> (x*y=w804:dbl)
              n514 = Insert Into Array(array=u16[] [] ("values"), index=0 ("索引"), new element=w804) -> (w808:u16[])
              n515 = case shown="真" w811 {
                tunnel: w808 -> [_ w823]
                tunnel: w807 -> [w817 w822]
                tunnel: [w817 w821] -> w803
                tunnel: [_ w820] -> w802
                tunnel: w801 -> [_ w819]
                frame False {
                }
                frame True {
                  n516 = Increment(x=w819) -> (x+1=→"当前校准":i32)
                  n517 = Bundle By Name(cluster=cluster{"starting address":u16, "values":u16[]} {"starting address"=4272, "values"=[]}, "starting address"=u16 4274, "values"=w823) -> (w825:cluster{"starting address":u16, "values":u16[]})
                  n518 = Enqueue Element(queue=w822, element=w825) -> (queue out=w821:refnum<queue>, error out=w820:errorcluster)  [unwired: 2 in, 1 out]
                }
              }
            }
          }
          frame #1 {
            n519 = local read "当前校准"() -> (w834:i32)
            n520 = case shown="5" w834 {
              tunnel: [w840 w841 w842 w843 w844] -> w833
              frame 1, Default {
                n521 = local read "浓度1"() -> (w840:dbl)
              }
              frame 2 {
                n522 = local read "浓度2"() -> (w841:dbl)
              }
              frame 3 {
                n523 = local read "浓度3"() -> (w842:dbl)
              }
              frame 4 {
                n524 = local read "浓度4"() -> (w843:dbl)
              }
              frame 5 {
                n525 = local read "浓度5"() -> (w844:dbl)
              }
            }
            n526 = Not Equal To 0?(x=w833) -> (x != 0?=w832:bool)
            n527 = case shown="假" w832 {
              tunnel: [u16 8 ("address") u16 9 ("address")] -> w837
              tunnel: ["校零" ("测量模式") "校标" ("测量模式")] -> w827
              frame False {
              }
              frame True {
              }
            }
            n528 = global write "COD测量模式全局.vi" "测量模式"(w827) -> ()
            n529 = Insert Into Array(array=u16[] [] ("values"), index=0 ("索引"), new element=w837) -> (w831:u16[])
            n530 = Bundle By Name(cluster=cluster{"starting address":u16, "values":u16[]} {"starting address"=0, "values"=[]}, "starting address"=u16 4608 ("address"), "values"=w831) -> (w839:cluster{"starting address":u16, "values":u16[]})
            n531 = Enqueue Element(queue=w829, element=w839, error in (no error)=w828) -> ()  [unwired: 1 in, 3 out]
          }
          frame #2 {
            n532 = local write "枚举"(enum16{"读取数据", "写入数据", "读取写入DATABASE", "读取参数"}."写入数据" ("枚举")) -> ()
            n533 = call <vilib>:"Application Directory.vi"() -> ("Application Directory"=w856:path)
            n534 = Build Path(base path=w856, name or relative path="data\\Set.ini" ("名称或相对路径")) -> (appended path=w858:path)
            n535 = local read "当前校准"() -> (w851:i32)
            n536 = call <vilib>:"Open Config Data.vi"("configuration file path"=w858) -> ("error out"=w854:errorcluster, "refnum"=w855:T10)  [unwired: 8 in, 1 out]
            n537 = call-poly <vilib>:"Write Key.vi"("section"="CODMn", "error in (no error)"=w854, "value"=w851, "key"="当前选用的校准" ("section"), "refnum"=w855) -> ("error out"=w849:errorcluster, "refnum out"=w850:T10)  [unwired: 4 in, 1 out]
            n538 = call <vilib>:"Close Config Data.vi"("error in (no error)"=w849, "refnum"=w850) -> ()  [unwired: 8 in, 2 out]
          }
        }
      }
      event "自动切换量程", "低切高阈值", "高切低阈值": Value Change {
        w864 = "CODMn是否切换量程" ("key")
        n539 = event-data() -> ()  [unwired: 1 in, 6 out]
        n540 = call <vilib>:"Application Directory.vi"() -> ("Application Directory"=w877:path)
        n541 = Build Path(base path=w877, name or relative path="data\\Set.ini" ("名称或相对路径")) -> (appended path=w875:path)
        n542 = local read "自动切换量程"() -> (w871:bool)
        n543 = call <vilib>:"Open Config Data.vi"("configuration file path"=w875) -> ("error out"=w873:errorcluster, "refnum"=w874:T10)  [unwired: 8 in, 1 out]
        n544 = call-poly <vilib>:"Write Key.vi"("section"=w864, "error in (no error)"=w873, "value"=w871, "key"="自动切换量程", "refnum"=w874) -> ("error out"=w867:errorcluster, "refnum out"=w868:T10)  [unwired: 4 in, 1 out]
        n545 = local read "低切高阈值"() -> (w863:dbl)
        n546 = call-poly <vilib>:"Write Key.vi"("section"=w864, "error in (no error)"=w867, "value"=w863, "key"="低切高阈值", "refnum"=w868) -> ("error out"=w865:errorcluster, "refnum out"=w866:T10)  [unwired: 4 in, 1 out]
        n547 = local read "高切低阈值"() -> (w862:dbl)
        n548 = call-poly <vilib>:"Write Key.vi"("section"=w864, "error in (no error)"=w865, "value"=w862, "key"="高切低阈值", "refnum"=w866) -> ("error out"=w860:errorcluster, "refnum out"=w861:T10)  [unwired: 4 in, 1 out]
        n549 = call <vilib>:"Close Config Data.vi"("error in (no error)"=w860, "refnum"=w861) -> ()  [unwired: 8 in, 2 out]
      }
      event "模型": Value Change {
        n550 = event-data() -> ()  [unwired: 1 in, 6 out]
        n551 = call <vilib>:"Application Directory.vi"() -> ("Application Directory"=w887:path)
        n552 = Build Path(base path=w887, name or relative path="data\\Set.ini" ("名称或相对路径")) -> (appended path=w885:path)
        n553 = call <vilib>:"Open Config Data.vi"("configuration file path"=w885) -> ("error out"=w883:errorcluster, "refnum"=w884:T10)  [unwired: 8 in, 1 out]
        n554 = local read "模型"() -> (w878:enum32{"线性", "多项式"})
        n555 = call-poly <vilib>:"Write Key.vi"("section"="CODMn模型选择" ("key"), "error in (no error)"=w883, "value"=w878, "key"="线性和多项式", "refnum"=w884) -> ("error out"=w879:errorcluster, "refnum out"=w880:T10)  [unwired: 4 in, 1 out]
        n556 = call <vilib>:"Close Config Data.vi"("error in (no error)"=w879, "refnum"=w880) -> ()  [unwired: 8 in, 2 out]
      }
      event "浓度1", "浓度2", "浓度3", "泵滴定数1", "泵滴定数2", "泵滴定数3", "启用1", "启用2", "启用3", "浓度4", "浓度5", "泵滴定数4", "泵滴定数5", "启用4", "启用5": Value Change {
        n557 = event-data() -> ()  [unwired: 1 in, 6 out]
        n558 = local read "选用水样"() -> (w903:enum16{"葡萄糖", "草酸钠"})
        n559 = local read "量程选择"() -> (w902:enum16{"低量程", "高量程", "0-2量程"})
        n560 = case shown="\"0-2量程\"" w902 {
          tunnel: ["低量程" "高量程" "0-2量程"] -> w900
          frame "低量程", Default {
          }
          frame "高量程" {
          }
          frame "0-2量程" {
          }
        }
        n561 = call <vilib>:"Application Directory.vi"() -> ("Application Directory"=w962:path)
        n562 = case shown="\"葡萄糖\", 默认" w903 {
          tunnel: ["葡萄糖标线" ("section") "草酸钠标线" ("section")] -> w909
          frame "葡萄糖", Default {
          }
          frame "草酸钠" {
          }
        }
        n563 = Build Path(base path=w962, name or relative path="data\\Set.ini" ("名称或相对路径")) -> (appended path=w960:path)
        n564 = call <vilib>:"Open Config Data.vi"("configuration file path"=w960) -> ("error out"=w958:errorcluster, "refnum"=w959:T10)  [unwired: 8 in, 1 out]
        n565 = local read "浓度1"() -> (w956:dbl)
        n566 = Concatenate Strings(w909, w900) -> (w901:string)
        n567 = local read "浓度2"() -> (w940:dbl)
        n568 = call-poly <vilib>:"Write Key.vi"("section"=w901, "error in (no error)"=w958, "value"=w956, "key"="浓度1", "refnum"=w959) -> ("error out"=w955:errorcluster, "refnum out"=w954:T10)  [unwired: 4 in, 1 out]
        n569 = local read "浓度3"() -> (w936:dbl)
        n570 = call-poly <vilib>:"Write Key.vi"("section"=w901, "error in (no error)"=w955, "value"=w940, "key"="浓度2", "refnum"=w954) -> ("error out"=w953:errorcluster, "refnum out"=w952:T10)  [unwired: 4 in, 1 out]
        n571 = local read "泵滴定数1"() -> (w934:dbl)
        n572 = call-poly <vilib>:"Write Key.vi"("section"=w901, "error in (no error)"=w953, "value"=w936, "key"="浓度3", "refnum"=w952) -> ("error out"=w951:errorcluster, "refnum out"=w950:T10)  [unwired: 4 in, 1 out]
        n573 = call-poly <vilib>:"Write Key.vi"("section"=w901, "error in (no error)"=w951, "value"=w934, "key"="泵滴定数1", "refnum"=w950) -> ("error out"=w949:errorcluster, "refnum out"=w948:T10)  [unwired: 4 in, 1 out]
        n574 = local read "泵滴定数2"() -> (w932:dbl)
        n575 = call-poly <vilib>:"Write Key.vi"("section"=w901, "error in (no error)"=w949, "value"=w932, "key"="泵滴定数2", "refnum"=w948) -> ("error out"=w947:errorcluster, "refnum out"=w946:T10)  [unwired: 4 in, 1 out]
        n576 = local read "泵滴定数3"() -> (w930:dbl)
        n577 = local read "浓度4"() -> (w899:dbl)
        n578 = call-poly <vilib>:"Write Key.vi"("section"=w901, "error in (no error)"=w947, "value"=w930, "key"="泵滴定数3", "refnum"=w946) -> ("error out"=w945:errorcluster, "refnum out"=w944:T10)  [unwired: 4 in, 1 out]
        n579 = local read "浓度5"() -> (w898:dbl)
        n580 = call-poly <vilib>:"Write Key.vi"("section"=w901, "error in (no error)"=w945, "value"=w899, "key"="浓度4", "refnum"=w944) -> ("error out"=w938:errorcluster, "refnum out"=w939:T10)  [unwired: 4 in, 1 out]
        n581 = call-poly <vilib>:"Write Key.vi"("section"=w901, "error in (no error)"=w938, "value"=w898, "key"="浓度5", "refnum"=w939) -> ("error out"=w896:errorcluster, "refnum out"=w897:T10)  [unwired: 4 in, 1 out]
        n582 = local read "泵滴定数4"() -> (w895:dbl)
        n583 = call-poly <vilib>:"Write Key.vi"("section"=w901, "error in (no error)"=w896, "value"=w895, "key"="泵滴定数4", "refnum"=w897) -> ("error out"=w943:errorcluster, "refnum out"=w942:T10)  [unwired: 4 in, 1 out]
        n584 = local read "泵滴定数5"() -> (w894:dbl)
        n585 = call-poly <vilib>:"Write Key.vi"("section"=w901, "error in (no error)"=w943, "value"=w894, "key"="泵滴定数5", "refnum"=w942) -> ("error out"=w892:errorcluster, "refnum out"=w893:T10)  [unwired: 4 in, 1 out]
        n586 = local read "启用1"() -> (w918:bool)
        n587 = call-poly <vilib>:"Write Key.vi"("section"=w901, "error in (no error)"=w892, "value"=w918, "key"="启用1", "refnum"=w893) -> ("error out"=w914:errorcluster, "refnum out"=w917:T10)  [unwired: 4 in, 1 out]
        n588 = local read "启用2"() -> (w915:bool)
        n589 = call-poly <vilib>:"Write Key.vi"("section"=w901, "error in (no error)"=w914, "value"=w915, "key"="启用2", "refnum"=w917) -> ("error out"=w925:errorcluster, "refnum out"=w924:T10)  [unwired: 4 in, 1 out]
        n590 = local read "启用3"() -> (w913:bool)
        n591 = call-poly <vilib>:"Write Key.vi"("section"=w901, "error in (no error)"=w925, "value"=w913, "key"="启用3", "refnum"=w924) -> ("error out"=w923:errorcluster, "refnum out"=w922:T10)  [unwired: 4 in, 1 out]
        n592 = local read "启用4"() -> (w888:bool)
        n593 = call-poly <vilib>:"Write Key.vi"("section"=w901, "error in (no error)"=w923, "value"=w888, "key"="启用4", "refnum"=w922) -> ("error out"=w921:errorcluster, "refnum out"=w920:T10)  [unwired: 4 in, 1 out]
        n594 = local read "启用5"() -> (w889:bool)
        n595 = call-poly <vilib>:"Write Key.vi"("section"=w901, "error in (no error)"=w921, "value"=w889, "key"="启用5", "refnum"=w920) -> ("error out"=w890:errorcluster, "refnum out"=w891:T10)  [unwired: 4 in, 1 out]
        n596 = local read "选用水样"() -> (w908:enum16{"葡萄糖", "草酸钠"})
        n597 = call-poly <vilib>:"Write Key.vi"("section"="标线选择", "error in (no error)"=w890, "value"=w908, "key"="选用水样", "refnum"=w891) -> ("error out"=w905:errorcluster, "refnum out"=w906:T10)  [unwired: 4 in, 1 out]
        n598 = call <vilib>:"Close Config Data.vi"("error in (no error)"=w905, "refnum"=w906) -> ()  [unwired: 8 in, 2 out]
      }
      event "读取": Value Change {
        n599 = event-data() -> ()  [unwired: 1 in, 6 out]
        n600 = local write "枚举"(enum16{"读取数据", "写入数据", "读取写入DATABASE", "读取参数"}."读取参数" ("枚举")) -> ()
        n601 = Bundle By Name(cluster=T5 {"starting address"=0, "number of holding registers"=0}, "starting address"=u16 4616, "number of holding registers"=u16 28) -> (w977:T5)
        n602 = Flush Queue(queue=w970, error in (no error)=w969) -> (queue out=w973:refnum<queue>, error out=w972:errorcluster)  [unwired: 1 out]
        n603 = Enqueue Element(queue=w973, element=w977, error in (no error)=w972) -> ()  [unwired: 1 in, 3 out]
        "读取KB值" <- TRUE
      }
      event "写入": Mouse Down {
        n604 = event-data() -> ()  [unwired: 1 in, 8 out]
        n605 = flat-sequence {
          tunnel: w978 -> [w981]
          frame #0 {
            n606 = local read "模型"() -> (w979:enum32{"线性", "多项式"})
            n607 = case shown="\"线性\", 默认" w979 {
              tunnel: [w993 w1000] -> w983
              tunnel: w981 -> [w987 w999]
              tunnel: [w987 w999] -> w980
              frame "线性", Default {
                n608 = local read "K"() -> (w990:dbl)
                n609 = local read "b"() -> (w989:dbl)
                n610 = Build Array(w990, w989, 0.0 ("元素")) -> (w988:dbl[])
                n611 = local read "量程选择"() -> (w986:enum16{"低量程", "高量程", "0-2量程"})
                n612 = call "浮点转CDAB整形cod.vi"("浮点数"=w988) -> ("CDAB整形输出"=w991:u16[])  [unwired: 10 in]
                n613 = case shown="\"0-2量程\"" w986 {
                  tunnel: [u16 4626 ("starting address") u16 4632 ("starting address") u16 4638 ("starting address")] -> w985
                  frame "低量程", Default {
                  }
                  frame "高量程" {
                  }
                  frame "0-2量程" {
                  }
                }
                n614 = Bundle By Name(cluster=cluster{"starting address":u16, "values":u16[]} {"starting address"=4272, "values"=[]}, "starting address"=w985, "values"=w991) -> (w993:cluster{"starting address":u16, "values":u16[]})
              }
              frame "多项式" {
                # "b,k,c"
                n615 = local read "多项式系数1"() -> (w1007:dbl[])
                n616 = local read "量程选择"() -> (w997:enum16{"低量程", "高量程", "0-2量程"})
                n617 = Index Array(array=w1007) -> (element #1=w1002:dbl, element #2=w1003:dbl, element #3=w998:dbl)  [unwired: 3 in]
                n618 = Build Array(w1003, w1002, w998) -> (w1006:dbl[])
                n619 = case shown="\"0-2量程\"" w997 {
                  tunnel: [u16 4626 ("starting address") u16 4632 ("starting address") u16 4638 ("starting address")] -> w1004
                  frame "低量程", Default {
                  }
                  frame "高量程" {
                  }
                  frame "0-2量程" {
                  }
                }
                n620 = call "浮点转CDAB整形cod.vi"("浮点数"=w1006) -> ("CDAB整形输出"=w1005:u16[])  [unwired: 10 in]
                n621 = Bundle By Name(cluster=cluster{"starting address":u16, "values":u16[]} {"starting address"=4272, "values"=[]}, "starting address"=w1004, "values"=w1005) -> (w1000:cluster{"starting address":u16, "values":u16[]})
              }
            }
            n622 = Enqueue Element(queue=w980, element=w983, timeout in ms (-1)=1000 ("超时毫秒(-1)")) -> ()  [unwired: 1 in, 3 out]
          }
          frame #1 {
            n623 = local write "枚举"(enum16{"读取数据", "写入数据", "读取写入DATABASE", "读取参数"}."写入数据" ("枚举")) -> ()
          }
        }
      }
      event "滴定曲线": Value Change {
        n624 = event-data() -> ()  [unwired: 1 in, 6 out]
        n625 = property on="窗格" class="Pane"("Origin"=T9 {"Horizontal"=0, "Vertical"=3200} ("原点")) -> ()  [unwired: 2 in, 2 out]
      }
      event "历史波形": Value Change {
        n626 = event-data() -> ()  [unwired: 1 in, 6 out]
        n627 = call-poly <vilib>:"Read Waveforms from File.vi"() -> ("error out"=w1013:errorcluster, "first waveform in record"=w1014:waveform(dbl))  [unwired: 6 in, 2 out]
        n628 = case shown="无错误" w1013 {
          tunnel: w1014 -> [w1017 _]
          frame No Error {
            n629 = Unbundle By Name(w1017) -> ("t0"=→"波形时间":timestamp, "Y"=w1016:dbl[])  [unwired: 2 out]
            n630 = local write "ORP滴定曲线2"(w1016) -> ()
            n631 = local write "滴定数-ORP值"(w1016) -> ()
          }
          frame Error {
            n632 = One Button Dialog(message="打开失败" ("消息")) -> ()  [unwired: 1 in, 1 out]
          }
        }
      }
    }
  }
  n633 = while {
    tunnel: w32 -> [w1148]
    tunnel: w31 -> [w1147]
    tunnel: w22 -> [w1143]
    tunnel: w21 -> [w1142]
    stop <- FALSE stop-if-true
    w1073 = T14 0 items=["最小二乘", "最小绝对残差", "Bisquare"] ("method")
    n634 = local read "浓度5"() -> (w1043:dbl)
    n635 = local read "浓度4"() -> (w1044:dbl)
    n636 = local read "浓度2"() -> (w1084:dbl)
    n637 = local read "浓度3"() -> (w1085:dbl)
    n638 = local read "浓度1"() -> (w1083:dbl)
    n639 = local read "泵滴定数3"() -> (w1088:dbl)
    n640 = Wait (ms)(milliseconds to wait=u32 500 ("等待时间（毫秒）")) -> ()  [unwired: 1 out]
    n641 = local read "泵滴定数2"() -> (w1087:dbl)
    n642 = local read "泵滴定数4"() -> (w1042:dbl)
    n643 = local read "泵滴定数5"() -> (w1041:dbl)
    n644 = local read "泵滴定数1"() -> (w1086:dbl)
    n645 = Bundle By Name(cluster=T5 {"starting address"=4224, "number of holding registers"=16}, "starting address"=u16 4224, "number of holding registers"=u16 50) -> (w1201:T5)
    n646 = local read "自动切换量程"() -> (w1039:bool)
    n647 = local read "基本量程"() -> (w1056:enum16{"10mg/L", "20mg/L"})
    n648 = Build Array("启用1", "启用2", "启用3", "启用4", "启用5") -> (w1031:bool[])
    n649 = Build Array(w1083, w1084, w1085, w1044, w1043) -> (w1075:dbl[])
    n650 = Build Array(w1086, w1087, w1088, w1042, w1041) -> (w1074:dbl[])
    n651 = Multiply(x="浓度 2", y=100.0) -> (x*y=w1123:dbl)
    n652 = Multiply(x="修正系数 2", y=100.0) -> (x*y=w1120:dbl)
    n653 = Select(t=T11."Enabled" ("禁用"), s=w1039, f=T11."Disabled and Grayed Out" ("禁用")) -> (s? t:f=w1037:T11)
    n654 = Multiply(x="温度", y=10.0) -> (x*y=w1126:dbl)
    n655 = global write "COD浓度全局变量.vi" "跨度液浓度"("跨度液浓度") -> ()
    n656 = call "线性公式CODMn用.vi"("标液浓度"=w1075, "监测浓度"=w1074, "启用"=w1031, "method"=w1073, "模型"="模型", "精度"=6) -> ("拟合方程"=→"拟合公式":string, "r^2"=→"r^2":dbl, "slope"=→"K":dbl, "intercept"=→"b":dbl, "XY图"=→"XY图":cluster{"X Values":dbl[], "Y Values":dbl[]}[], "Polynomial Coefficients"=→"多项式系数1":dbl[])  [unwired: 8 in]
    n657 = global write "COD浓度全局变量.vi" "基本量程"(w1056) -> ()
    n658 = local write "修正系数"(w1120) -> ()
    n659 = local write "温度 2"(w1126) -> ()
    n660 = property on="低切高阈值" class="DigNum (严格)"("DisabledEnum"=w1037) -> ()  [unwired: 2 in, 2 out]
    n661 = property on="高切低阈值" class="DigNum (严格)"("DisabledEnum"=w1037) -> ()  [unwired: 2 in, 2 out]
    n662 = local write "浓度"(w1123) -> ()
    n663 = disable-structure shown="禁用" {
      frame Disabled {
        n664 = global read "系统变量.vi" "自动切换量程"() -> (w1235:bool)
        n665 = local write "自动切换量程"(w1235) -> ()
      }
      frame Enabled {
      }
    }
    n666 = Enqueue Element(queue=w1148, element=w1201, error in (no error)=w1147) -> ()  [unwired: 1 in, 3 out]
    n667 = local read "Registers"() -> (w1065:u16[])
    n668 = To Word Integer(number=w1065) -> (16bit integer=w1064:i16[])
    n669 = Index Array(array=w1064, index #1=0 ("索引"), index #4=3 ("索引"), index #14=13 ("索引"), index #15=14 ("索引"), index #32=31 ("索引")) -> (element #1=w1117:i16, element #2=w1116:i16, element #3=w1115:i16, element #4=w1030:i16, element #5=→"模式（受控）":i16, element #6=→"进样管":i16, element #7=→"高锰酸钾":i16, element #8=→"草酸钠":i16, element #9=→"硫酸":i16, element #10=w1063:i16, element #11=w1175:i16, element #12=w1026:i16, element #13=w1055:i16, element #14=w1192:i16, element #15=w1150:i16, element #16=w1029:i16, element #33=→"分":i16, element #34=→"秒":i16)  [unwired: 29 in, 16 out]
    "多列列表框" <- w1029
    n670 = Build Array(w1117, w1116, w1115) -> (w1118:i16[])
    n671 = To Single Precision Float(number=w1063) -> (single precision float=→"ORP显示":sgl)
    n672 = Divide(x=w1150, y=u16 1000) -> (x/y=→"标度滴定值":dbl)
    n673 = Divide(x=w1175, y=u16 10) -> (x/y=→"温度":dbl)
    n674 = Equal?(x=w1026, y=u16 2) -> (x = y?=→"断电排液标记":bool)
    n675 = global write "COD测量模式全局.vi" "CODMn工作状态"(w1030) -> ()
    n676 = Equal?(x=w1055, y=u16 2) -> (x = y?=w1053:bool)
    "温控器故障" <- w1053
    n677 = Equal?(x=w1055, y=u16 3) -> (x = y?=w1052:bool)
    "加热故障" <- w1052
    n678 = Equal?(x=w1055, y=u16 4) -> (x = y?=w1051:bool)
    "高锰酸钾报警" <- w1051
    n679 = Equal?(x=w1055, y=u16 5) -> (x = y?=w1050:bool)
    "草酸钠报警" <- w1050
    n680 = Equal?(x=w1055, y=u16 6) -> (x = y?=w1049:bool)
    "测量错误" <- w1049
    n681 = Equal?(x=w1055, y=u16 8) -> (x = y?=w1048:bool)
    "校零错误" <- w1048
    n682 = Equal?(x=w1055, y=u16 7) -> (x = y?=w1047:bool)
    "校标错误" <- w1047
    n683 = Equal?(x=w1055, y=u16 9) -> (x = y?=w1046:bool)
    "进水样超量程" <- w1046
    n684 = Divide(x=w1192, y=u16 1000) -> (x/y=→"零点滴定值":dbl)
    n685 = Equal?(x=w1055, y=u16 10) -> (x = y?=w1045:bool)
    "排液故障" <- w1045
    n686 = Equal?(x=w1026, y=u16 1) -> (x = y?=→"排液标记":bool)
    n687 = global write "运行时序全局变量.vi" "多列列表框"(w1029) -> ()
    n688 = Equal?(x=w1055, y=u16 1) -> (x = y?=w1054:bool)
    "ORP故障" <- w1054
    n689 = Equal?(x=w1030, y=u16 0) -> (x = y?=→"待机":bool)
    n690 = Equal?(x=w1030, y=u16 8) -> (x = y?=→"校零标记":bool)
    n691 = Equal?(x=w1030, y=u16 9) -> (x = y?=→"校标标记":bool)
    n692 = Equal?(x=w1030, y=u16 1) -> (x = y?=→"水样测量":bool)
    n693 = Equal?(x=w1030, y=u16 7) -> (x = y?=→"质控样测量":bool)
    n694 = Equal?(x=w1030, y=u16 10) -> (x = y?=→"加标回收测量":bool)
    n695 = Equal?(x=w1030, y=u16 2) -> (x = y?=→"标样核查标记":bool)
    n696 = Equal?(x=w1030, y=u16 6) -> (x = y?=→"平行样测量":bool)
    n697 = Equal?(x=w1030, y=u16 3) -> (x = y?=→"零点核查标记":bool)
    n698 = Equal?(x=w1030, y=u16 4) -> (x = y?=→"跨度核查标记":bool)
    n699 = Equal?(x=w1030, y=u16 5) -> (x = y?=→"空白测试标记":bool)
    n700 = feedback #2(w1029) -> (w1133:i16)
    n701 = feedback-in #2(w1029) -> ()
    n702 = Compound Arithmetic op=OR ("复合运算")(w1054, w1053, w1052, w1051, w1050, w1049, w1047, w1048, w1046, w1045) -> (→"故障标记":bool)
    n703 = Not Equal?(x=w1029, y=w1133) -> (x != y?=w1132:bool)
    n704 = Bundle By Name(cluster=T3 {"ORP故障"=FALSE, "温控器故障"=FALSE, "加热故障"=FALSE, "高锰酸钾报警"=FALSE, "草酸钠报警"=FALSE, "测量错误"=FALSE, "校零错误"=FALSE, "校标错误"=FALSE, " 进水样超量程"=FALSE, "排液阀故障"=FALSE} ("报警簇"), "ORP故障"=w1054, "温控器故障"=w1053, "加热故障"=w1052, "高锰酸钾报警"=w1051, "草酸钠报警"=w1050, "测量错误"=w1049, "校零错误"=w1048, "校标错误"=w1047, "进水样超量程"=w1046, "排液阀故障"=w1045) -> (w1134:T3)
    "报警簇" <- w1134
    n705 = local read "断电排液标记"() -> (w1024:bool)
    n706 = call "HexToDate.vi"("数组"=w1118) -> ("DATE"=w1113:timestamp[])  [unwired: 10 in]
    n707 = Index Array(array=w1113) -> (element=→"仪器时间":timestamp)  [unwired: 1 in]
    n708 = First Call?() -> (First Call?: T/F=w1022:bool)
    n709 = Get Date/Time In Seconds() -> (seconds since 1Jan1904=w1112:timestamp)
    "系统时间" <- w1112
    n710 = call <vilib>:"Boolean Crossing PtByPt.vi"("direction"=enum16{"either", "false-true", "true-false"}."false-true", "input"=w1024) -> ("crossing"=w1023:bool)  [unwired: 1 in]
    n711 = call "CODMn报警信息.vi"("报警簇"=w1134) -> ("CODMN报警信息"=w1135:string)  [unwired: 10 in]
    n712 = case shown="假" w1022 {
      tunnel: w1132 -> [w1206 _]
      tunnel: w1029 -> [w1205 _]
      frame False {
        n713 = case shown="真" w1206 {
          tunnel: w1205 -> [_ w1218]
          frame False {
          }
          frame True {
            n714 = property on="多列列表框" class="MCListbox (严格)"() -> ("ItemNames"=w1212:string[][])  [unwired: 2 in, 2 out]
            n715 = Index Array(array=w1212, index (row)=w1218) -> (element=w1209:string[])  [unwired: 1 in]
            n716 = Index Array(array=w1209, index=0 ("索引")) -> (element=w1207:string)
            n717 = Array To Spreadsheet String(delimiter (Tab)="-" ("分隔符(Tab)"), array=w1209, 3:"" ("格式字符串")) -> ()  [unwired: 1 out]
            n718 = Get Date/Time In Seconds() -> (seconds since 1Jan1904=w1216:timestamp)
            n719 = Bundle(cluster=T12 {"时间标识"=timestamp(0 s since 1904-01-01), "参数"="", "日志信息"="", "流程参数"=""} ("data in"), "时间标识"=w1216, "参数"="CODMn" ("table输入"), "日志信息"=w1207, "流程参数"="" ("table输入")) -> (w1213:T12)
            n720 = call "流程日志字段定义.vi"("table输入"="操作日志", "data in"=w1213) -> ("table输出"=w1221:string, "columns"=w1222:string[], "data out"=w1223:T15)  [unwired: 7 in]
            n721 = call "插入数据.vi"("data"=w1223, "columns"=w1222, "database"="database3.mdb", "table"=w1221) -> ()  [unwired: 7 in, 1 out]
          }
        }
      }
      frame True {
      }
    }
    n722 = Less Or Equal?(x=w1029, y=u16 4) -> (x <= y?=w1081:bool)
    n723 = case shown="真" w1023 {
      frame False {
      }
      frame True {
        n724 = Get Date/Time In Seconds() -> (seconds since 1Jan1904=w1229:timestamp)
        n725 = Bundle(cluster=T12 {"时间标识"=timestamp(0 s since 1904-01-01), "参数"="", "日志信息"="", "流程参数"=""} ("data in"), "时间标识"=w1229, "参数"="CODMn" ("table输入"), "日志信息"="断电排液", "流程参数"="" ("table输入")) -> (w1227:T12)
        n726 = call "流程日志字段定义.vi"("table输入"="操作日志", "data in"=w1227) -> ("table输出"=w1232:string, "columns"=w1233:string[], "data out"=w1234:T15)  [unwired: 7 in]
        n727 = call "插入数据.vi"("data"=w1234, "columns"=w1233, "database"="database3.mdb", "table"=w1232) -> ()  [unwired: 7 in, 1 out]
      }
    }
    n728 = Equal?(x=w1029, y=u16 5) -> (x = y?=w1146:bool)
    n729 = feedback #3(w1135) -> (w1136:string)
    n730 = feedback-in #3(w1135) -> ()
    n731 = Greater?(x=w1029, y=u16 0) -> (0:w1078:bool)
    n732 = Not Equal?(x=w1135, y="") -> (x != y?=w1140:bool)
    n733 = case shown="真" w1081 {
      frame False {
      }
      frame True {
        n734 = local read "测量模式数字"() -> (w1245:i32)
        n735 = local read "标样核查标记"() -> (w1248:bool)
        n736 = local read "零点核查标记"() -> (w1247:bool)
        n737 = local read "跨度核查标记"() -> (w1243:bool)
        n738 = local read "空白测试标记"() -> (w1242:bool)
        n739 = local read "加标回收测量"() -> (w1241:bool)
        n740 = local read "平行样测量"() -> (w1240:bool)
        n741 = local read "启动时间"() -> (w1237:timestamp)
        n742 = local read "水样测量"() -> (w1249:bool)
        n743 = local read "校零标记"() -> (w1239:bool)
        n744 = local read "校标标记"() -> (w1238:bool)
        n745 = case shown="0, 默认" w1245 {
          tunnel: ["水样测试" ("测量模式") "标样核查" ("测量模式") "零点核查" ("测量模式") "跨度核查" ("测量模式") "空白测试" ("测量模式") "加标回收" ("测量模式") "平行样" ("测量模式") "校零" ("测量模式") "校标" ("测量模式")] -> w1244
          tunnel: w1237 -> [w1250 _ _ _ _ w1256 _ _ _]
          frame 0, Default {
            n746 = global write "COD测量模式全局.vi" "水样启动时间"(w1250) -> ()
          }
          frame 1 {
          }
          frame 2 {
          }
          frame 3 {
          }
          frame 4 {
          }
          frame 5 {
            n747 = global write "COD测量模式全局.vi" "加标回收启动时间"(w1256) -> ()
          }
          frame 6 {
          }
          frame 7 {
          }
          frame 8 {
          }
        }
        n748 = Build Array(w1249, w1248, w1247, w1243, w1242, w1241, w1240, w1239, w1238) -> (w1246:bool[])
        n749 = for {
          tunnel: w1246 -> [w1262] mode=indexing
          i -> [w1261]
          n750 = case shown="真" w1262 {
            tunnel: w1261 -> [_ w1263]
            frame False {
            }
            frame True {
              "测量模式数字" <- w1263
            }
          }
        }
        n751 = global write "COD测量模式全局.vi" "测量模式"(w1244) -> ()
      }
    }
    n752 = global read "COD读取DATA全局.vi" "data"() -> (w1096:T16)
    n753 = call <vilib>:"Boolean Crossing PtByPt.vi"("direction"=enum16{"either", "false-true", "true-false"}."false-true", "input"=w1146) -> ("crossing"=w1144:bool)  [unwired: 1 in]
    n754 = call <vilib>:"Boolean Crossing PtByPt.vi"("direction"=enum16{"either", "false-true", "true-false"}."false-true", "input"=w1078) -> ("crossing"=w1077:bool)  [unwired: 1 in]
    n755 = Build Array(w1112) -> (w1111:timestamp[])
    n756 = Not Equal?(x=w1135, y=w1136) -> (x != y?=w1137:bool)
    n757 = case shown="真" w1144 {
      tunnel: w1143 -> [_ w1316]
      tunnel: w1142 -> [_ w1311]
      frame False {
      }
      frame True {
        n758 = Bundle By Name(cluster=T5 {"starting address"=0, "number of holding registers"=0}, "starting address"=u16 4101, "number of holding registers"=u16 10) -> (w1315:T5)
        n759 = Enqueue Element(queue=w1316, element=w1315, error in (no error)=w1311) -> ()  [unwired: 1 in, 3 out]
        n760 = local write "枚举"(enum16{"读取数据", "写入数据", "读取写入DATABASE", "读取参数"}."读取写入DATABASE" ("枚举")) -> ()
      }
    }
    n761 = case shown="真" w1077 {
      frame False {
      }
      frame True {
        n762 = Get Date/Time In Seconds() -> (seconds since 1Jan1904=→"启动时间":timestamp)
      }
    }
    n763 = global read "COD测量模式全局.vi" "测量模式"() -> (w1095:string)
    n764 = call "DateToHex.vi"("DATE"=w1111) -> ("数组"=w1110:u16[])  [unwired: 10 in]
    n765 = call "DateToHex.vi"("DATE"=w1113) -> ("数组"=w1105:u16[])  [unwired: 10 in]
    n766 = And(x=w1137, y=w1140) -> (x .and. y?=w1138:bool)
    n767 = Unbundle By Name(w1096) -> ("时间"=w1093:timestamp, "检测值"=w1092:sgl, "数据标识"=w1091:string)
    n768 = case shown="真" w1138 {
      tunnel: w1135 -> [_ w1300]
      frame False {
      }
      frame True {
        n769 = Get Date/Time In Seconds() -> (seconds since 1Jan1904=w1302:timestamp)
        n770 = Bundle By Name(cluster=T13 {"时间标识"=timestamp(0 s since 1904-01-01), "设备"="", "日志信息"=""} ("data in"), "时间标识"=w1302, "设备"="CODMn", "日志信息"=w1300) -> (w1303:T13)
        n771 = call "报警信息字段定义.vi"("table输入"="报警信息", "data in"=w1303) -> ("table输出"=w1307:string, "columns"=w1308:string[], "data out"=w1309:T13)  [unwired: 7 in]
        n772 = call "插入数据.vi"("data"=w1309, "columns"=w1308, "database"="database3.mdb", "table"=w1307) -> ()  [unwired: 7 in, 1 out]
      }
    }
    n773 = Index Array(array=w1105, index=2 ("索引")) -> (element=w1107:u16)
    n774 = Index Array(array=w1110, index=2 ("索引")) -> (element=w1108:u16)
    n775 = local read "测量数据区"() -> (w1097:T2)
    n776 = case shown="\"水样测试\"" w1095 {
      tunnel: w1097 -> [w1264 w1269 w1274 w1279 w1284 w1289 w1294 w1299]
      tunnel: [w1264 w1268 w1270 w1278 w1283 w1288 w1290 w1298] -> w1094
      tunnel: w1093 -> [_ w1267 w1273 w1277 w1282 w1287 w1293 w1297]
      tunnel: w1092 -> [_ w1266 w1272 w1276 w1281 w1286 w1292 w1296]
      tunnel: w1091 -> [_ w1265 w1271 w1275 w1280 w1285 w1291 w1295]
      frame "", Default {
      }
      frame "水样测试" {
        n777 = Bundle By Name(cluster=w1269, "水样数据时间"=w1267, "水样实测值"=w1266, "水样数据标识"=w1265) -> (w1268:T2)
      }
      frame "标样核查" {
        n778 = Bundle By Name(cluster=w1274, "跨度核查数据时间"=w1273, "跨度核查实测值"=w1272, "跨度核查数据标识"=w1271) -> (w1270:T2)
      }
      frame "零点核查" {
        n779 = Bundle By Name(cluster=w1279, "零点核查数据时间"=w1277, "零点核查实测值"=w1276, "零点核查数据标识"=w1275) -> (w1278:T2)
      }
      frame "加标回收" {
        n780 = Bundle By Name(cluster=w1284, "加标回收数据时间"=w1282, "加标回收实测值"=w1281, "加标回收数据标识"=w1280) -> (w1283:T2)
      }
      frame "平行样" {
        n781 = Bundle By Name(cluster=w1289, "平行样数据时间"=w1287, "平行样实测值"=w1286, "平行样数据标识"=w1285) -> (w1288:T2)
      }
      frame "校零" {
        n782 = Bundle By Name(cluster=w1294, "空白数据时间"=w1293, "空白实测值"=w1292, "空白数据标识"=w1291) -> (w1290:T2)
      }
      frame "校标" {
        n783 = Bundle By Name(cluster=w1299, "标样数据时间"=w1297, "标样实测值"=w1296, "标样数据标识"=w1295) -> (w1298:T2)
      }
    }
    "测量数据区" <- w1094
    n784 = Split Number(x=w1107) -> (hi(x)=w1101:u8)  [unwired: 1 out]
    n785 = Split Number(x=w1108) -> (hi(x)=w1104:u8)  [unwired: 1 out]
    n786 = To Byte Integer(number=w1101) -> (8bit integer=w1100:i8)
    n787 = To Byte Integer(number=w1104) -> (8bit integer=w1103:i8)
    n788 = Subtract(x=w1100, y=w1103) -> (x-y=w1102:i8)
    n789 = local read "通讯状态"() -> (w1020:bool)
    n790 = Absolute Value(x=w1102) -> (abs(x)=w1099:i8)
    n791 = Greater Or Equal?(x=w1099, y=i8 1) -> (x >= y?=w1021:bool)
    n792 = And(x=w1021, y=w1020) -> (x .and. y?=w1019:bool)
    n793 = case shown="真" w1019 {
      frame False {
      }
      frame True {
        n794 = flat-sequence {
          frame #0 {
            n795 = property on="时间校准" class="Bool (严格)"("Val(Sgnl)"=TRUE ("值(信号)")) -> ()  [unwired: 2 in, 2 out]
          }
          frame #1 {
            n796 = Wait (ms)(milliseconds to wait=u32 500 ("等待时间（毫秒）")) -> ()  [unwired: 1 out]
          }
          frame #2 {
            n797 = property on="时间校准" class="Bool (严格)"("Val(Sgnl)"=FALSE ("值(信号)")) -> ()  [unwired: 2 in, 2 out]
          }
        }
      }
    }
  }
  n798 = while {
    tunnel: w2 -> [w1333]
    tunnel: w1 -> [w1332]
    tunnel: w18 -> [w1331]
    tunnel: w32 -> [w1330]
    tunnel: w31 -> [w1329]
    tunnel: [w1319] -> w30
    tunnel: [w1328] -> w29
    tunnel: w15 -> [w1326]
    tunnel: w14 -> [w1325]
    tunnel: w22 -> [w1324]
    tunnel: w21 -> [w1323]
    tunnel: w20 -> [w1322]
    tunnel: w18 -> [w1317]
    stop <- FALSE stop-if-true
    n799 = case shown="\"读取写入DATABASE\"" "枚举" {
      tunnel: w1333 -> [w1369 w1380 w1463 w1554]
      tunnel: w1332 -> [w1368 w1376 w1462 w1553]
      tunnel: w1331 -> [_ w1379 _ _]
      tunnel: [w1336 w1378 w1465 w1548] -> w1328
      tunnel: [w1335 w1377 w1464 w1546] -> w1319
      tunnel: w1330 -> [w1366 _ _ _]
      tunnel: w1329 -> [w1362 _ _ _]
      tunnel: w1326 -> [_ _ _ w1552]
      tunnel: w1325 -> [_ _ _ w1551]
      tunnel: w1324 -> [_ _ w1461 _]
      tunnel: w1323 -> [_ _ w1460 _]
      tunnel: w1322 -> [_ w1375 _ _]
      tunnel: w1317 -> [_ _ w1426 _]
      frame "读取数据", Default {
        n800 = Dequeue Element(queue=w1366, timeout in ms (-1)=1000 ("超时毫秒(-1)"), error in (no error)=w1362) -> (element=w1365:T5)  [unwired: 3 out]
        n801 = Unbundle By Name(w1365) -> ("starting address"=w1364:u16, "number of holding registers"=w1363:u16)
        n802 = call <vilib>:"Read Holding Registers.vi"("error in (no error)"=w1368, "quantity"=w1363, "starting address"=w1364, "MB session in"=w1369) -> ("error out"=w1334:errorcluster, "Registers"=w1367:u16[], "MB session out"=w1360:refnum<class "MB_Master_Serial.lvclass">)  [unwired: 5 in]
        n803 = case shown="无错误" w1334 {
          tunnel: w1367 -> [w1370 _]
          frame No Error {
            "Registers" <- w1370
          }
          frame Error {
          }
        }
        n804 = call <vilib>:"Read Coils.vi"("error in (no error)"=w1334, "quantity"=u16 8, "starting address"=u16 140, "MB session in"=w1360) -> ("error out"=w1348:errorcluster, "Coils"=w1357:bool[], "MB session out"=w1349:refnum<class "MB_Master_Serial.lvclass">)  [unwired: 5 in]
        n805 = Index Array(array=w1357) -> (element #1=→"进水样":bool, element #2=→"进蒸馏水":bool, element #3=→"进标液":bool, element #4=→"进质控样":bool, element #5=→"进加标回收样":bool, element #6=→"进高锰酸钾":bool, element #7=→"进草酸钠":bool, element #8=→"进硫酸":bool)  [unwired: 9 in, 1 out]
        n806 = call <vilib>:"Read Coils.vi"("error in (no error)"=w1348, "quantity"=u16 1, "starting address"=u16 137, "MB session in"=w1349) -> ("error out"=w1344:errorcluster, "Coils"=w1338:bool[], "MB session out"=w1345:refnum<class "MB_Master_Serial.lvclass">)  [unwired: 5 in]
        n807 = Index Array(array=w1338) -> (element=→"搅拌":bool)  [unwired: 1 in]
        n808 = call <vilib>:"Read Coils.vi"("error in (no error)"=w1344, "quantity"=u16 1, "starting address"=u16 400, "MB session in"=w1345) -> ("error out"=w1335:errorcluster, "Coils"=w1341:bool[], "MB session out"=w1336:refnum<class "MB_Master_Serial.lvclass">)  [unwired: 5 in]
        n809 = Index Array(array=w1341) -> (element=→"加热":bool)  [unwired: 1 in]
      }
      frame "写入数据" {
        n810 = flat-sequence {
          tunnel: w1380 -> [w1391]
          tunnel: w1379 -> [w1390]
          tunnel: w1376 -> [w1384]
          tunnel: w1375 -> [w1383]
          tunnel: [w1386] -> w1374
          tunnel: [w1385] -> w1373
          tunnel: [w1382] -> w1372
          tunnel: [w1381] -> w1371
          tunnel: [w1392] -> w1377
          tunnel: [w1398] -> w1378
          tunnel: w1374 -> [w1398]
          tunnel: w1373 -> [w1392]
          tunnel: w1372 -> [w1397]
          tunnel: w1371 -> [w1396]
          frame #0 {
            n811 = Dequeue Element(queue=w1390, error in (no error)=w1383) -> (queue out=w1382:refnum<queue>, element=w1389:cluster{"starting address":u16, "values":u16[]}, error out=w1381:errorcluster)  [unwired: 1 in, 1 out]
            n812 = Unbundle By Name(w1389) -> ("starting address"=w1388:u16, "values"=w1387:u16[])
            n813 = call <vilib>:"Write Multiple Registers.vi"("error in (no error)"=w1384, "values"=w1387, "starting address"=w1388, "MB session in"=w1391) -> ("error out"=w1385:errorcluster, "MB session out"=w1386:refnum<class "MB_Master_Serial.lvclass">)  [unwired: 6 in]
          }
          frame #1 {
            n814 = Get Queue Status(queue=w1397, error in (no error)=w1396) -> (# elements in queue=w1395:i32)  [unwired: 1 in, 7 out]
            n815 = Equal To 0?(x=w1395) -> (x = 0?=w1394:bool)
            n816 = case shown="真" w1394 {
              tunnel: [enum16{"读取数据", "写入数据", "读取写入DATABASE", "读取参数"}."写入数据" ("枚举") enum16{"读取数据", "写入数据", "读取写入DATABASE", "读取参数"}."读取数据" ("枚举")] -> w1393
              tunnel: w1392 -> [_ w1400]
              frame False {
              }
              frame True {
                n817 = case shown="无错误" w1400 {
                  tunnel: ["保存成功" ("消息") "保存失败" ("消息")] -> _
                  frame No Error {
                  }
                  frame Error {
                  }
                }
              }
            }
            n818 = local write "枚举"(w1393) -> ()
          }
        }
      }
      frame "读取写入DATABASE" {
        # "高量程0-5之间会乘1.2的系数\n低量程0-2之间会乘1.1的系数"
        n819 = Dequeue Element(queue=w1461, timeout in ms (-1)=1000 ("超时毫秒(-1)"), error in (no error)=w1460) -> (element=w1468:T5)  [unwired: 3 out]
        n820 = Unbundle By Name(w1468) -> ("starting address"=w1467:u16, "number of holding registers"=w1466:u16)
        n821 = call <vilib>:"Read Holding Registers.vi"("error in (no error)"=w1462, "quantity"=w1466, "starting address"=w1467, "MB session in"=w1463) -> ("error out"=w1464:errorcluster, "Registers"=w1410:u16[], "MB session out"=w1465:refnum<class "MB_Master_Serial.lvclass">)  [unwired: 5 in]
        n822 = To Word Integer(number=w1410) -> (16bit integer=w1409:i16[])
        n823 = Split 1D Array(array=w1409, index=3 ("索引")) -> (first subarray=w1458:i16[], second subarray=w1448:i16[])
        n824 = global read "系统变量.vi" "运行模式"() -> (w1429:enum16{"维护模式", "常规模式", "应急模式", "质控模式"})
        n825 = case shown="\"维护模式\", 默认" w1429 {
          tunnel: ["M" ("单位") "N" ("单位") "N" ("单位") "N" ("单位")] -> w1428
          frame "维护模式", Default {
          }
          frame "常规模式" {
          }
          frame "应急模式" {
          }
          frame "质控模式" {
          }
        }
        n826 = Index Array(array=w1458) -> (element #1=w1456:i16, element #2=w1455:i16, element #3=w1454:i16)  [unwired: 3 in]
        n827 = Index Array(array=w1448) -> (element #1=w1417:i16, element #2=w1452:i16, element #3=w1451:i16, element #4=w1450:i16, element #5=w1449:i16)  [unwired: 5 in]
        n828 = Index Array(array=w1448, index=6 ("索引")) -> (element=w1446:i16)
        n829 = To Single Precision Float(number=w1417) -> (single precision float=w1419:sgl)
        n830 = Divide(x=w1419, y=sgl 100.0) -> (x/y=w1418:sgl)
        n831 = Less Or Equal?(x=w1418, y=sgl 0.01) -> (x <= y?=w1421:bool)
        n832 = case shown="真" w1421 {
          tunnel: [w1537 w1538] -> w1420
          tunnel: w1418 -> [w1537 _]
          frame False {
          }
          frame True {
            n833 = Random Number (0-1)() -> (number: 0 to 1=w1541:dbl)
            n834 = Increment(x=w1541) -> (x+1=w1539:dbl)
            n835 = Divide(x=w1539, y=sgl 100.0) -> (x/y=w1538:dbl)
          }
        }
        n836 = Build Array(w1456, w1455, w1454) -> (w1453:i16[])
        n837 = To Single Precision Float(number=w1452) -> (single precision float=w1433:sgl)
        n838 = To Single Precision Float(number=w1446) -> (single precision float=w1423:sgl)
        n839 = To Single Precision Float(number=w1451) -> (single precision float=w1434:sgl)
        n840 = To Single Precision Float(number=w1450) -> (single precision float=w1435:sgl)
        n841 = To Single Precision Float(number=w1449) -> (single precision float=w1443:sgl)
        n842 = call "HexToDate.vi"("数组"=w1453) -> ("DATE"=w1457:timestamp[])  [unwired: 10 in]
        n843 = Index Array(array=w1457) -> (element=w1405:timestamp)  [unwired: 1 in]
        n844 = disable-structure shown="启用" {
          disable-tunnel: w1420 -> [w1470 w1494]
          disable-tunnel: [w1469 w1494] -> w1404
          frame Disabled {
            n845 = property on="基本量程" class="Enum (严格)"() -> ("Value"=w1471:enum16{"10mg/L", "20mg/L"})  [unwired: 2 in, 2 out]
            n846 = case shown="\"10mg/L\", 默认" w1471 {
              tunnel: w1470 -> [w1474 w1484]
              tunnel: [w1472 w1483] -> w1469
              frame "10mg/L", Default {
                n847 = Less Or Equal?(x=w1474, y=2.0) -> (x <= y?=w1477:bool)
                n848 = Greater?(x=w1474, y=0.0) -> (0:w1476:bool)
                n849 = And(x=w1477, y=w1476) -> (x .and. y?=w1473:bool)
                n850 = case shown="真" w1473 {
                  tunnel: w1474 -> [w1479 w1482]
                  tunnel: [w1479 w1480] -> w1472
                  frame False {
                  }
                  frame True {
                    n851 = Multiply(x=w1482, y=1.1) -> (x*y=w1480:dbl)
                  }
                }
              }
              frame "20mg/L" {
                n852 = Greater?(x=w1484, y=0.0) -> (0:w1487:bool)
                n853 = Less Or Equal?(x=w1484, y=5.0) -> (x <= y?=w1488:bool)
                n854 = And(x=w1488, y=w1487) -> (x .and. y?=w1485:bool)
                n855 = case shown="真" w1485 {
                  tunnel: w1484 -> [w1490 w1493]
                  tunnel: [w1490 w1491] -> w1483
                  frame False {
                  }
                  frame True {
                    n856 = Multiply(x=w1493, y=1.2) -> (x*y=w1491:dbl)
                  }
                }
              }
            }
          }
          frame Enabled {
          }
        }
        "COD浓度（mg/L)" <- w1404
        n857 = local write "启动时间"(w1405) -> ()
        n858 = Format Date/Time String(seconds (now)=w1405) -> (date/time string=→"数据时间":string)  [unwired: 2 in]
        n859 = global read "COD测量模式全局.vi" "测量模式"() -> (w1408:string)
        n860 = global read "COD测量模式全局.vi" "测量模式"() -> (w1424:string)
        n861 = global read "COD测量模式全局.vi" "测量模式"() -> (w1416:string)
        n862 = case shown="\"跨度核查\"" w1408 {
          tunnel: [0.0 w1496 w1499] -> w1407
          frame "", Default {
          }
          frame "标样核查", "校标" {
            n863 = local read "标样浓度 2"() -> (w1497:dbl)
            n864 = Divide(x=w1497, y=100.0) -> (x/y=w1496:dbl)
          }
          frame "跨度核查" {
            n865 = local read "跨度液浓度"() -> (w1499:dbl)
          }
        }
        n866 = Divide(x=w1443, y=sgl 1000.0) -> (x/y=w1436:sgl)
        n867 = Not Equal?(x=w1416, y="校标") -> (x != y?=w1414:bool)
        n868 = case shown="真" w1414 {
          tunnel: w1426 -> [_ w1510]
          tunnel: w1404 -> [_ w1508]
          frame False {
            n869 = local write "枚举"(enum16{"读取数据", "写入数据", "读取写入DATABASE", "读取参数"}."读取数据" ("枚举")) -> ()
          }
          frame True {
            n870 = case shown="真" "自动切换量程" {
              tunnel: w1510 -> [_ w1512]
              tunnel: w1508 -> [_ w1513]
              frame False {
                n871 = local write "枚举"(enum16{"读取数据", "写入数据", "读取写入DATABASE", "读取参数"}."读取数据" ("枚举")) -> ()
              }
              frame True {
                n872 = local read "基本量程"() -> (w1514:enum16{"10mg/L", "20mg/L"})
                n873 = case shown="\"20mg/L\"" w1514 {
                  tunnel: w1513 -> [w1517 w1529]
                  tunnel: w1512 -> [w1515 w1526]
                  frame "10mg/L", Default {
                    n874 = Greater?(x=w1517, y="低切高阈值") -> (0:w1516:bool)
                    n875 = case shown="真" w1516 {
                      tunnel: w1515 -> [_ w1520]
                      frame False {
                        n876 = local write "枚举"(enum16{"读取数据", "写入数据", "读取写入DATABASE", "读取参数"}."读取数据" ("枚举")) -> ()
                      }
                      frame True {
                        n877 = local write "枚举"(enum16{"读取数据", "写入数据", "读取写入DATABASE", "读取参数"}."写入数据" ("枚举")) -> ()
                        n878 = Bundle By Name(cluster=cluster{"starting address":u16, "values":u16[]} {"starting address"=0, "values"=[]}, "starting address"=u16 4276, "values"=u16[] [1]) -> (w1522:cluster{"starting address":u16, "values":u16[]})
                        n879 = Enqueue Element(queue=w1520, element=w1522) -> ()  [unwired: 2 in, 3 out]
                      }
                    }
                  }
                  frame "20mg/L" {
                    n880 = Less?(x=w1529, y="高切低阈值") -> (x < y?=w1527:bool)
                    n881 = case shown="真" w1527 {
                      tunnel: w1526 -> [_ w1531]
                      frame False {
                        n882 = local write "枚举"(enum16{"读取数据", "写入数据", "读取写入DATABASE", "读取参数"}."读取数据" ("枚举")) -> ()
                      }
                      frame True {
                        n883 = local write "枚举"(enum16{"读取数据", "写入数据", "读取写入DATABASE", "读取参数"}."写入数据" ("枚举")) -> ()
                        n884 = Bundle By Name(cluster=cluster{"starting address":u16, "values":u16[]} {"starting address"=0, "values"=[]}, "starting address"=u16 4276, "values"=u16[] [0]) -> (w1533:cluster{"starting address":u16, "values":u16[]})
                        n885 = Enqueue Element(queue=w1531, element=w1533) -> ()  [unwired: 2 in, 3 out]
                      }
                    }
                  }
                }
              }
            }
          }
        }
        n886 = local read "温度"() -> (w1427:dbl)
        n887 = Format Into String(format string="w%05d" ("格式字符串"), u32 1019 ("因子编码")) -> (resulting string=w1432:string)  [unwired: 2 in, 1 out]
        n888 = Bundle(cluster=T16 {"时间"=timestamp(0 s since 1904-01-01), "测量模式"="", "数据类型"="", "检测值"=0.0, "单位"="", "数据标识"="", "因子编码"="", "标样参考值"=0.0, "ORP-A"=0.0, "ORP-B"=0.0, "ORP-K"=0.0, "COD滴定值"=0.0, "高锰酸钾滴定数"=0.0, "温度"=0.0} ("data"), "时间"=w1405, "测量模式"=w1424, "数据类型"=w1428, "检测值"=w1404, "单位"="mg/L", "数据标识"="N", "因子编码"=w1432, "标样参考值"=w1407, "ORP-A"=w1433, "ORP-B"=w1434, "ORP-K"=w1435, "COD滴定值"=w1436, "高锰酸钾滴定数"=w1423, "温度"=w1427) -> (w1425:T16)
        n889 = global read "COD测量模式全局.vi" "测量模式"() -> (w1413:string)
        n890 = global write "COD浓度全局变量.vi" "COD浓度（mg/L)"(w1404) -> ()
        n891 = Equal?(x=w1413, y="校标") -> (x = y?=w1411:bool)
        n892 = global write "COD读取DATA全局.vi" "data"(w1425) -> ()
        n893 = case shown="真" w1411 {
          tunnel: w1423 -> [_ w1500]
          frame False {
          }
          frame True {
            n894 = local read "当前校准"() -> (w1501:i32)
            n895 = case shown="3" w1501 {
              tunnel: w1500 -> [w1502 w1503 w1504 w1505 w1506]
              frame 1, Default {
                n896 = local write "泵滴定数1"(w1502) -> ()
              }
              frame 2 {
                n897 = local write "泵滴定数2"(w1503) -> ()
              }
              frame 3 {
                n898 = local write "泵滴定数3"(w1504) -> ()
              }
              frame 4 {
                n899 = local write "泵滴定数4"(w1505) -> ()
              }
              frame 5 {
                n900 = local write "泵滴定数5"(w1506) -> ()
              }
            }
          }
        }
        n901 = call "存数据cloumns(子VI).vi"() -> ("数组"=w1441:string[])  [unwired: 11 in]
        n902 = call "数据写入database.vi"("data"=w1425, "columns"=w1441, "table"="CODMn") -> ()  [unwired: 8 in, 1 out]
      }
      frame "读取参数" {
        n903 = Dequeue Element(queue=w1552, timeout in ms (-1)=1000 ("超时毫秒(-1)"), error in (no error)=w1551) -> (element=w1558:T5)  [unwired: 3 out]
        n904 = local write "枚举"(enum16{"读取数据", "写入数据", "读取写入DATABASE", "读取参数"}."读取数据" ("枚举")) -> ()
        n905 = Unbundle By Name(w1558) -> ("starting address"=w1557:u16, "number of holding registers"=w1556:u16)
        n906 = local read "读取KB值"() -> (w1547:bool)
        n907 = call <vilib>:"Read Holding Registers.vi"("error in (no error)"=w1553, "quantity"=w1556, "starting address"=w1557, "MB session in"=w1554) -> ("error out"=w1546:errorcluster, "Registers"=w1550:u16[], "MB session out"=w1548:refnum<class "MB_Master_Serial.lvclass">)  [unwired: 5 in]
        n908 = case shown="假" w1547 {
          tunnel: w1550 -> [w1568 w1593]
          tunnel: w1546 -> [_ w1595]
          frame False {
            n909 = Index Array(array=w1568) -> (element #1=w1562:u16, element #2=w1581:u16, element #3=w1580:u16, element #4=w1560:u16, element #5=w1579:u16, element #6=w1578:u16, element #7=w1577:u16, element #8=w1576:u16, element #9=w1575:u16, element #10=w1574:u16, element #11=w1573:u16, element #12=w1572:u16, element #13=w1571:u16, element #14=w1570:u16, element #15=w1569:u16, element #16=w1567:u16)  [unwired: 16 in]
            n910 = local write "浓度"(w1580) -> ()
            n911 = local write "水样"(w1578) -> ()
            n912 = local write "硫酸"(w1571) -> ()
            n913 = local write "标液"(w1576) -> ()
            n914 = Divide(x=w1562, y=u16 10) -> (x/y=w1563:dbl)
            n915 = local write "草酸钠"(w1572) -> ()
            n916 = local write "蒸馏水"(w1577) -> ()
            n917 = local write "质控样"(w1575) -> ()
            n918 = local write "恒温时间"(w1581) -> ()
            n919 = local write "基本量程"(w1579) -> ()
            n920 = local write "加标回收"(w1574) -> ()
            n921 = local write "高锰酸钾"(w1573) -> ()
            n922 = local write "零点泵计量数 2"(w1570) -> ()
            n923 = local write "标度泵计量数 2"(w1569) -> ()
            n924 = Divide(x=w1560, y=u16 100) -> (x/y=w1559:dbl)
            n925 = Divide(x=w1567, y=u16 100) -> (x/y=w1566:dbl)
            n926 = local write "温度"(w1563) -> ()
            n927 = local write "修正系数 2"(w1559) -> ()
            n928 = local write "浓度 2"(w1566) -> ()
          }
          frame True {
            (unwired) 9 ("索引")
            n929 = case shown="错误" w1595 {
              tunnel: ["读取成功" ("消息") "读取失败" ("消息")] -> w1594
              frame No Error {
              }
              frame Error {
              }
            }
            n930 = Array Subset(array=w1593, index=10 ("索引"), length=18 ("长度")) -> (w1590:u16[])
            n931 = call "浮点CDAB转换COD.vi"("数组"=w1590) -> ("数组 2"=w1589:sgl[])  [unwired: 10 in]
            n932 = One Button Dialog(message=w1594) -> ()  [unwired: 1 in, 1 out]
            n933 = Array To Cluster(array=w1589) -> (cluster=w1588:T17)
            n934 = local read "量程选择"() -> (w1582:enum16{"低量程", "高量程", "0-2量程"})
            n935 = case shown="\"0-2量程\"" w1582 {
              tunnel: w1588 -> [w1599 w1603 w1607]
              tunnel: [w1598 w1602 w1606] -> w1585
              tunnel: [w1597 w1601 w1605] -> w1584
              tunnel: [w1596 w1600 w1604] -> w1583
              frame "低量程", Default {
                n936 = Unbundle By Name(w1599) -> ("数组 2[2]"=w1598:sgl, "数组 2[0]"=w1597:sgl, "数组 2[1]"=w1596:sgl)
              }
              frame "高量程" {
                n937 = Unbundle By Name(w1603) -> ("数组 2[5]"=w1602:sgl, "数组 2[3]"=w1601:sgl, "数组 2[4]"=w1600:sgl)
              }
              frame "0-2量程" {
                n938 = Unbundle By Name(w1607) -> ("数组 2[8]"=w1606:sgl, "数组 2[6]"=w1605:sgl, "数组 2[7]"=w1604:sgl)
              }
            }
            n939 = Bundle By Name(cluster=cluster{"X^2":dbl, "X":dbl, "b":dbl} {"X^2"=0.0, "X"=0.0, "b"=0.0} ("方程系数"), "X^2"=w1585, "X"=w1584, "b"=w1583) -> (w1586:cluster{"X^2":dbl, "X":dbl, "b":dbl})
            n940 = local write "方程系数"(w1586) -> ()
          }
        }
      }
    }
    n941 = Unbundle By Name(w1319) -> ("status"=w1320:bool)
    n942 = Not(x=w1320) -> (.not. x?=→"通讯状态":bool)
  }
  n943 = call-dynamic "Close Session.vi"("error in (no error)"=w30, "MB_Serial session"=w29) -> ()  [unwired: 9 in, 1 out]
  "COM" <- "VISA resource name"
